vi "Control Experiment.vi"(8 "Error In":errorcluster, 9 "KH":T5={"KH #"=[0, 1, 2, 3, 4, 5, 6, 7, 8, 9, 10, 11, 12, 13, 14, 15], "KH Configuration"=[enum."SE+ (-gnd)", enum."SE+ (-gnd)", enum."Differential", enum."Differential", enum."SE+ (-gnd)", enum."Differential", enum."Differential", enum."SE+ (-gnd)", enum."Differential", enum."Differential", enum."SE+ (-gnd)", enum."SE+ (-gnd)", enum."Differential", enum."Ground", enum."Ground", enum."Ground"], "KH Gain"=[enum."1000x", enum."1000x", enum."1000x", enum."1000x", enum."1000x", enum."1000x", enum."1000x", enum."1000x", enum."1000x", enum."1000x", enum."1000x", enum."1000x", enum."1000x", enum."1000x", enum."1000x", enum."100x"], "KH Shunt Resistor"=[enum."Open", enum."Open", enum."Open", enum."5k Ohms", enum."Open", enum."Open", enum."5k Ohms", enum."Open", enum."Open", enum."5k Ohms", enum."Open", enum."Open", enum."50k Ohms", enum."Open", enum."Open", enum."Open"]}, 10 "Lockin":T7={"AI"=[1, 2, 3, 4, 5, 6, 7, 8, 9, 10, 11, 12, 13, 14, 15, 16], "Electrode"=["4", "5", "6", "7", "9", "11", "12", "13", "16", "17", "20", "21", "1", "", "", ""], "Label"=[12, 14, 15, 13, 10, 11, 9, 8, 4, 2, 1, 3, 6, 0, 0, 0], "Electrode Config"=[enum."Current", enum."Voltage (SE)", enum."Voltage (SE)", enum."Current", enum."Voltage (SE)", enum."Voltage (SE)", enum."Current", enum."Current", enum."Voltage (SE)", enum."Current", enum."Current", enum."Voltage (SE)", enum."Gate", enum."Voltage (SE)", enum."Voltage (SE)", enum."Voltage (SE)"]} {"Label" items=["", "I+", "I-", "V1+", "V1-", "dV1", "Vsg", "Vbg", "I2+", "I2-", "V2+", "V2-", "I3+", "I3-", "V3+", "V3-"]}) -> (0 "Error Out":errorcluster)   [LabVIEW 2019, in "Control Experiment.lvclass"]
doc: "Use this VI to help configure your experiment.\n1. Choose Pickering or Not Pickering\n2. Configure the Electrode control to show which electrode is connected to which lockin\n3. Choose a Label for each electrode to configure Krohn Hite amplifier automatically\n4. Easily set all Krohn Hite channels to be \"all ground\" or \"all differential\" mode\n5. Fill out information about you and your device in the lower left corner\n6. When you are finished, or when you want to update the amplifiers, click the \"CREATE OUTPUT\" button located in upper right. Clicking this button will set the amplifiers, Pickering switch (if you have one), and write information to a functional global variable that you can easily read from elsewhere in your program"
uses:
  Control Experiment.lvclass
  Typedefs/Instrument--enum.ctl
  <userlib>/LevyLab/Krohn Hite 7008/typedefs/Shunt-Enum.ctl
  Typedefs/KH Mode-enum.ctl
  <userlib>/LevyLab/Krohn Hite 7008/typedefs/Input Configuration-Enum.ctl
  <userlib>/LevyLab/Krohn Hite 7008/typedefs/Gain-Enum.ctl
  <userlib>/LevyLab/Krohn Hite 7008/typedefs/SetAll-Array.ctl
  <userlib>/LevyLab/Krohn Hite 7008/typedefs/SetAll-Cluster.ctl
  <userlib>/LevyLab/Krohn Hite 7008/typedefs/Channel-Enum.ctl
  <userlib>/LevyLab/Krohn Hite 7008/typedefs/Filter-Enum.ctl
  <userlib>/LevyLab/Krohn Hite 7008/typedefs/Coupling-Enum.ctl
  <userlib>/LevyLab/Instrument Framework/SMOs/Configuration/Configuration.lvclass
  Typedefs/UI Controls --cluster.ctl
  <userlib>/LevyLab/Instrument Framework/SMOs/Logger.PGSQL/Logger.PGSQL.lvclass
  C:/Program Files (x86)/National Instruments/LabVIEW 2019/vi.lib/JKI/JKI SMO/SMO/SMO.lvclass
  Control Experiment.lvclass/Control Experiment.ctl
  <userlib>/_MGI/File/MGI Create Directory Chain Behavior Enum.ctl
  Typedefs/Control Experiment JSON--cluster.ctl
  <userlib>/LevyLab/Krohn Hite 7008/Instrument.KH7008.lvclass/Instrument.KH7008.ctl
  23189d07-d529-447d-957d-13a42bf56e57.vi
  9a447b37-f4f5-4836-8e27-fdda23b4a061.vi
  <vilib>/JDP Science/JSONtext/Variant to JSON Text.vi
  <vilib>/regexp/Match Regular Expression.xnode
  <vilib>/JDP Science/JSONtext/LVClass Serializer/JSONtext LVClass Serializer.lvclass
  <userlib>/LevyLab/Krohn Hite 7008/Instrument.KH7008.lvclass
  <vilib>/JKI/JKI SMO/SMO/SMO.lvclass
  <userlib>/LevyLab/Lockin-Multichannel/Instrument.Lockin/Instrument.Lockin.lvclass
panel:
  out "KH Addresses":refnum<visa-resource-name>[](array[refnum])=["COM20", "COM14"] caption="KH Address[A,B,C,...]"
  in  "I'm Finished Taking Data!":bool
  out "Values have changed":bool=TRUE
  in  "Create Output":bool
  in  "OK":bool
  out "Control Experiment":refnum<class "Control Experiment.lvclass">
  in  "C.E.":refnum<class "Control Experiment.lvclass">
  in  "Tab Control":T1(tab)
  in  "Instrument Configuration":bool
  out "Instruments":string="    devices:\n    \n    1. 80x80um rectangle\n    2. hash: 200 horizontal and vertical lines 400nm apart\n    3. hash structures: 400, 200nm apart horizontal and vertical lines"
  in  "DC Coupled":bool=TRUE
  in  "Bandwidth Filter":bool=TRUE
  in  "AO Channels":u32=8
  in  "Gain":dbl[](array[numeric])=[1.0, 1.0, 1.0, 1.0, 1.0, 1.0, 1.0, 1.0, 1.0, 1.0, 1.0, 1.0, 1.0, 1.0, 1.0, 1.0]
  in  "AI Channels":u32=16
  in  "KH All Buttons":T8(radio)
  in  "Defualt Shunt Resistor":T4=enum."5k Ohms"
  in  "Description":string="    devices:\n    \n    1. 80x80um rectangle\n    2. hash: 200 horizontal and vertical lines 400nm apart\n    3. hash structures: 400, 200nm apart horizontal and vertical lines"
  in  "Sample (SAXXXX)":string="SA40178"
  in  "Device (YYYYMMDD)":string="20210125"
  in  "Instrument":T9=enum."MNK"
  in  "Username":string="Aditi"
  in  "non KH":T10 {"Labels 2" items=["", "I+", "I-", "V1+", "V1-", "dV1", "Vsg", "Vbg", "I2+", "I2-", "V2+", "V2-", "I3+", "I3-", "V3+", "V3-"]}
  in  "Ring":u16(ring)=2 items=["----Sweep Control----", "Sweep Control.vi", "Continuous B Sweep.vi", "----Transport----", "IV.vi", "IV_Sweep.vi", "Lockin_time.vi", "Lockin_Vsg.vi", "Lockin_sweep.vi", "Lockin_AIWFM_time.vi", "THz_TimeDelay.vi", "Sweep_AIWFM_time.vi"]
  in  "Open VI":bool
  in  "Open Lockin":bool
  in  "Default Path":path=path "C:/temp" caption="Default Path (Do not add your instrument name here)(Typ. G:\\My Drive\\ansom\\Data)"
  out "Comments":string="Device: \r  Device Name: SA40178.20210125\r  Computer: KHOLEK\r  User: Aditi\r  Instrument: MNK\r  Description: |\r        devices:\r        \r        1. 80x80um rectangle\r        2. hash: 200 horizontal and vertical lines 400nm apart\r        3. hash structures: 400, 200nm apart horizontal and vertical lines\r\rExperiment: \r  Time: 2021-02-22T11:02:02\r  Description: |\r\rSweep: \r- Loop1: [OFF, 0.000000]\r- Loop2: [OFF, 0.000000]\r- Loop3: [OFF, 0.000000]\r- Loop4: [OFF, 0.000000]\r\rWiring: \r- Electrode 4: Lockin 1, V2, KH1 Channel 1, SE+ (-gnd), 1000x, Open\r- Electrode 5: Lockin 2, V2, KH1 Channel 2, SE+ (-gnd), 1000x, Open\r- Electrode 6: Lockin 3, I2, KH1 Channel 3, Differential, 1000x, 5k Ohms\r- Electrode 7: Lockin 4, I2, KH1 Channel 4, Differential, 1000x, 5k Ohms\r- Electrode 9: Lockin 5, V2, KH1 Channel 5, SE+ (-gnd), 1000x, Open\r- Electrode 11: Lockin 6, I2, KH1 Channel 6, Differential, 1000x, 5k Ohms\r- Electrode 12: Lockin 7, I2, KH1 Channel 7, Differential, 1000x, 5k Ohms\r- Electrode 13: Lockin 8, V2, KH1 Channel 8, SE+ (-gnd), 1000x, Open\r- Electrode 16: Lockin 9, I-, KH2 Channel 1, Differential, 1000x, 5k Ohms\r- Electrode 17: Lockin 10, I+, KH2 Channel 2, Differential, 1000x, 5k Ohms\r- Electrode 20: Lockin 11, V1+, KH2 Channel 3, SE+ (-gnd), 1000x, Open\r- Electrode 21: Lockin 12, V1-, KH2 Channel 4, SE+ (-gnd), 1000x, Open\r- Electrode 1: Lockin 13, Vsg, KH2 Channel 5, Differential, 1000x, 50k Ohms\r\rLockin: \r  AO: \r  - AO 1: amp = 0.000 mV, DC = 0.000 mV, f = 1.00 Hz, phi = 0.00°, Triangle\r  - AO 2: amp = 0.000 mV, DC = 0.000 mV, f = 1.00 Hz, phi = 0.00°, Triangle\r  - AO 3: amp = 0.000 mV, DC = 0.000 mV, f = 1.00 Hz, phi = 0.00°, Triangle\r  - AO 4: amp = 0.000 mV, DC = 0.000 mV, f = 1.00 Hz, phi = 0.00°, Triangle\r  - AO 5: amp = 0.000 mV, DC = 0.000 mV, f = 1.00 Hz, phi = 0.00°, Triangle\r  - AO 6: amp = 10.000 mV, DC = 0.000 mV, f = 1.00 Hz, phi = 0.00°, Triangle\r  - AO 7: amp = 0.000 mV, DC = 0.000 mV, f = 1.00 Hz, phi = 0.00°, Triangle\r  - AO 8: amp = 0.000 mV, DC = 0.000 mV, f = 1.00 Hz, phi = 0.00°, Triangle\r  - AO 9: amp = 0.000 mV, DC = 0.000 mV, f = 1.00 Hz, phi = 0.00°, Triangle\r  - AO 10: amp = 10.000 mV, DC = 0.000 mV, f = 1.00 Hz, phi = 0.00°, Triangle\r  - AO 11: amp = 0.000 mV, DC = 0.000 mV, f = 1.00 Hz, phi = 0.00°, Triangle\r  - AO 12: amp = 0.000 mV, DC = 0.000 mV, f = 1.00 Hz, phi = 0.00°, Triangle\r  - AO 13: amp = 0.000 mV, DC = 0.000 mV, f = 1.00 Hz, phi = 0.00°, Sine\r  - AO 14: amp = 0.000 mV, DC = 0.000 mV, f = 1.00 Hz, phi = 0.00°, Sine\r  - AO 15: amp = 0.000 mV, DC = 0.000 mV, f = 1.00 Hz, phi = 0.00°, Sine\r  - AO 16: amp = 0.000 mV, DC = 0.000 mV, f = 1.00 Hz, phi = 0.00°, Sine\r  - AO 17: amp = 0.000 mV, DC = -0.000 mV, f = 1.00 Hz, phi = 0.00°, Sine\r  - AO 18: amp = 0.000 mV, DC = 0.000 mV, f = 1.00 Hz, phi = 0.00°, Sine\r  - AO 19: amp = 0.000 mV, DC = 0.000 mV, f = 1.00 Hz, phi = 0.00°, Sine\r  - AO 20: amp = 0.000 mV, DC = 0.000 mV, f = 1.00 Hz, phi = 0.00°, Sine\r  - AO 21: amp = 0.000 mV, DC = 0.000 mV, f = 1.00 Hz, phi = 0.00°, Sine\r  - AO 22: amp = 0.000 mV, DC = 0.000 mV, f = 1.00 Hz, phi = 0.00°, Sine\r  - AO 23: amp = 0.000 mV, DC = 0.000 mV, f = 1.00 Hz, phi = 0.00°, Sine\r  - AO 24: amp = 0.000 mV, DC = 0.000 mV, f = 1.00 Hz, phi = 0.00°, Sine\r  REF: \r  - Lockin 1: f = 1.00 Hz, phi = 0.00°, TC = 0.10 s, order = 2 \r  Sampling: \r  - Fs: 10000.000000\r  - N: 1000\r"
  out "Device Folder":path=path "D:/Data/MNK/SA40178.20210125" caption="(\\base path\\project\\device\\ )"
  out "JSON String":string="{\r\n    \"Device\":{\r\n        \"Device\":\"SA40178.20210125\",\r\n        \"User\":\"Aditi\",\r\n        \"Time\":\"2021-02-22T11:02:02\",\r\n        \"Computer Name\":\"KHOLEK\"\r\n    },\r\n    \"Wiring\":{\r\n        \"Lockin Ch\":[\r\n            1,\r\n            2,\r\n            3,\r\n            4,\r\n            5,\r\n            6,\r\n            7,\r\n            8,\r\n            9,\r\n            10,\r\n            11,\r\n            12,\r\n            13,\r\n            14,\r\n            15,\r\n            16\r\n        ],\r\n        \"KH Electrodes\":[\r\n            \"4\",\r\n            \"5\",\r\n            \"6\",\r\n            \"7\",\r\n            \"9\",\r\n            \"11\",\r\n            \"12\",\r\n            \"13\",\r\n            \"16\",\r\n            \"17\",\r\n            \"20\",\r\n            \"21\",\r\n            \"1\",\r\n            \"\",\r\n            \"\",\r\n            \"\"\r\n        ],\r\n        \"KH Labels\":[\r\n            \"V2\",\r\n            \"V2\",\r\n            \"I2\",\r\n            \"I2\",\r\n            \"V2\",\r\n            \"I2\",\r\n            \"I2\",\r\n            \"V2\",\r\n            \"I-\",\r\n            \"I+\",\r\n            \"V1+\",\r\n            \"V1-\",\r\n            \"Vsg\",\r\n            \"\",\r\n            \"\",\r\n            \"\"\r\n        ],\r\n        \"Other Electrodes\":[\r\n            \"4\",\r\n            \"5\",\r\n            \"6\",\r\n            \"7\",\r\n            \"9\",\r\n            \"11\",\r\n            \"12\",\r\n            \"13\",\r\n            \"16\",\r\n            \"17\",\r\n            \"20\",\r\n            \"21\",\r\n            \"1\",\r\n            \"\",\r\n            \"\",\r\n            \"\"\r\n        ],\r\n        \"Other Labels\":[\r\n            \"V2\",\r\n            \"V2\",\r\n            \"I2\",\r\n            \"I2\",\r\n            \"V2\",\r\n            \"I2\",\r\n            \"I2\",\r\n            \"V2\",\r\n            \"I-\",\r\n            \"I+\",\r\n            \"V1+\",\r\n            \"V1-\",\r\n            \"Vsg\",\r\n            \"\",\r\n            \"\",\r\n            \"\"\r\n        ]\r\n    }\r\n}"
  in  "Labels Strings":string[](array[string])=["", "I+", "I-", "V1+", "V1-", "dV1", "Vsg", "Vbg", "I2+", "I2-", "V2+", "V2-", "I3+", "I3-", "V3+", "V3-"]
  out "YAML example":string="description: This is a dummy dataset which mimics smFRET data.\n\nsetup:\n    ## Mandatory fields\n    num_pixels: 2                # using 2 detectors\n    num_spots: 1                 # a single confocal excitation\n    num_spectral_ch: 2           # donor and acceptor detection\n    num_polarization_ch: 1       # no polarization selection\n    num_split_ch: 1              # no beam splitter\n    modulated_excitation: False  # CW excitation, no modulation\n    lifetime: False              # no TCSPC in detection\n\n    ## Optional fields\n    excitation_wavelengths:      # List of excitation wavelenghts\n       - !!float 532e-9\n    excitation_cw:               # List of booleans, True if wavelength is CW\n       - True\n    detection_wavelengths:       # Nominal center wavelength for each for detection ch\n       - !!float 580e-9\n       - !!float 640e-9\n\nsample:\n  sample_name: describe the sample here\n  buffer_name: describe the buffer here\n  dye_names: 'Cy3B, ATTO647N'   # Comma separates names of fluorophores\n\nidentity:\n    author: Author Name\n    author_affiliation: Name of Research Institution\n\nprovenance:\n    filename: 'photon_data.hdf5'\n    software: Acquisition Software Name\n\nphoton_data:\n    timestamps_specs:\n        timestamps_unit: !!float 10e-9  # 10 ns\n    measurement_specs:\n        measurement_type: smFRET\n        detectors_specs:\n            spectral_ch1: [0]  # list of donor's detector IDs\n            spectral_ch2: [1]  # list of acceptor's detector IDs"
  in  "String":string
  # "SANDBOX:"
  # "Sample"
  # "Krohn Hite"
  # "Lockin"
  # "Lockin"
  # "Krohn Hite"
  # "Other"
  # "Device and Project Description"
  # "Instrument Configuration"
  # "Experiment VIs"
  # "Path Configuration"
  # "Use this VI to help configure your experiment.\n1. Configure the Electrode control to show which electrode is connected to which lockin\n2. Choose a Label for each electrode to configure Krohn Hite amplifier automatically\n3. Easily set all Krohn Hite channels to be \"all ground\" or \"all differential\" mode\n4. Fill out information about you and your device in the lower left corner\n5. When you are finished, or when you want to update the amplifiers, click the \"CREATE OUTPUT\" button located in upper right.\nClicking this button will set the amplifiers, Pickering switch (if you have one), and write information to a functional global variable that you can easily read from elsewhere in your program"
  # "If you want to have new labels for the \"Labels\" field you can type them here"
  # "The magic words are:\nI\nVsg\nVbg\ndV\nV"
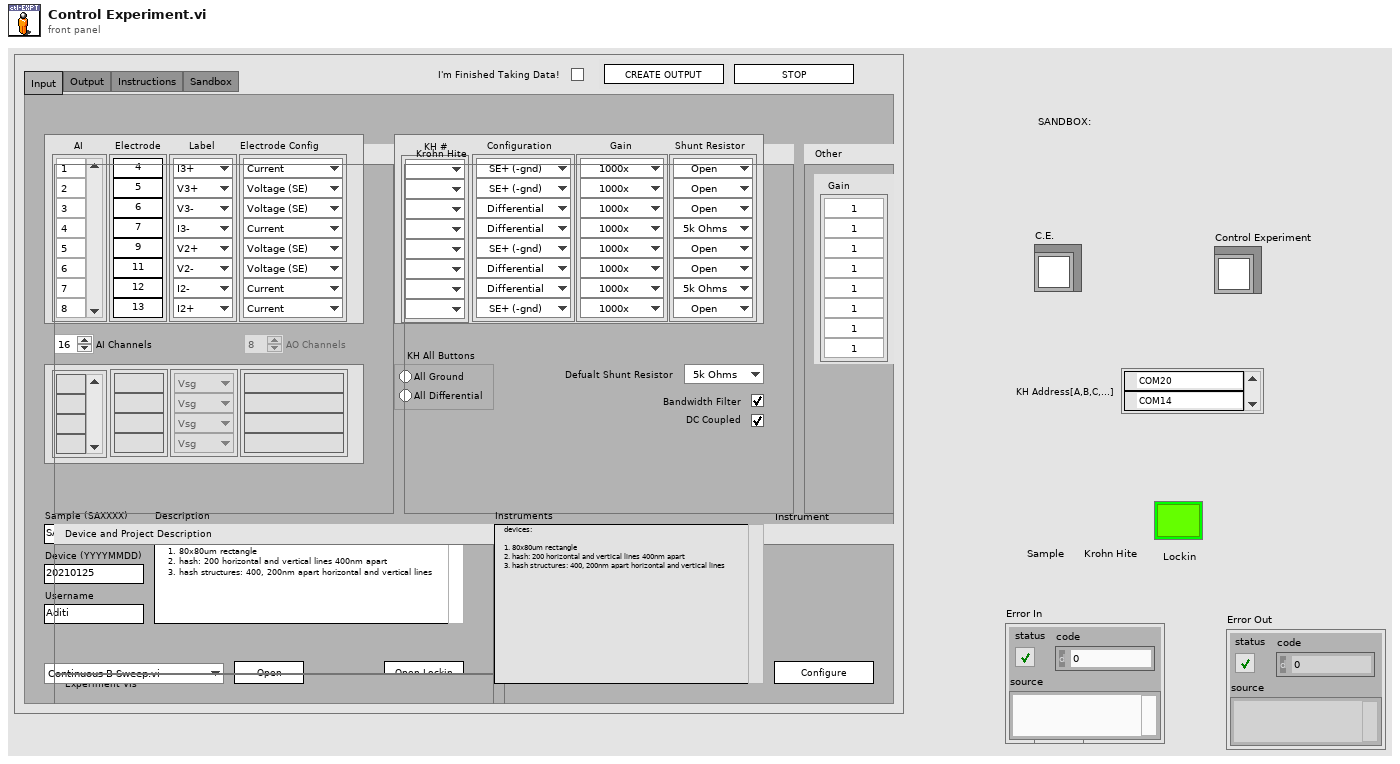
[diagram p1: front panel]
types:
  T1 = enum32{"Input", "Output", "Instructions", "Sandbox"}
  T2 = typedef "Instrument.KH7008.lvclass/Input Configuration-Enum.ctl" = enum16{"Ground", "SE+ (-gnd)", "SE- (+gnd)", "Differential"}
  T3 = typedef "Instrument.KH7008.lvclass/Gain-Enum.ctl" = enum16{"1x", "10x", "100x", "1000x"}
  T4 = typedef "Instrument.KH7008.lvclass/Shunt-Enum.ctl" = enum16{"Open", "50 Ohms", "500 Ohms", "5k Ohms", "50k Ohms", "10M Ohm"}
  T5 = cluster{"KH #":u16[], "KH Configuration":T2[], "KH Gain":T3[], "KH Shunt Resistor":T4[]}
  T6 = typedef "Control Experiment.lvclass/KH Mode-enum.ctl" = enum16{"Ground", "Current", "Voltage (SE)", "Voltage (Diff)", "Gate"}
  T7 = cluster{"AI":u32[], "Electrode":string[], "Label":u16[], "Electrode Config":T6[]}
  T8 = enum32{"No Selection", "All Ground", "All Differential"}
  T9 = typedef "Control Experiment.lvclass/Instrument--enum.ctl" = enum16{"----- AFM/EBL -----", "AGILENT", "CYPHER", "Gemini2", "JEOL", "MFP3D", "----- Cryostat -----", "CF900", "DR200", "MNK", "PPMS (simulated)", "PPMS 1", "PPMS 2", "PPMS 3", "----- Optics -----", "THz 1 (Element 2/Montana)", "THz 2 (Tsunami/Janis)"}
  T10 = cluster{"Scroll Bar":string[], "Electrodes 2":string[], "Labels 2":u16[], "unused":string[]}
  T11 = enum32{"invalid app kind", "Development System", "Run Time System", "Student Edition", "Embedded LabVIEW", "Evaluation", "Custom"}
  T12 = enum32{"Bad", "Idle", "Run top level", "Running"}
  T13 = enum32{"Invalid", "Standard", "Closed", "Hidden", "Minimized", "Maximized"}
  T14 = typedef "MGI Create Directory Chain Behavior Enum.ctl" = enum16{"Auto Detect", "Path Contains a File", "Path Does Not Contain a File"}
  T15 = typedef "Instrument.KH7008.lvclass/SetAll-Cluster.ctl" = cluster{"Channel":T16, "Gain":T3, "Bandwidth Filter":T17, "Shunt Resistor":T4, "Coupling":T18, "Input Config":T2}
  T16 = typedef "Instrument.KH7008.lvclass/Channel-Enum.ctl" = enum16{"Channel 1", "Channel 2", "Channel 3", "Channel 4", "Channel 5", "Channel 6", "Channel 7", "Channel 8"}
  T17 = typedef "Instrument.KH7008.lvclass/Filter-Enum.ctl" = enum16{"OFF", "ON"}
  T18 = typedef "Instrument.KH7008.lvclass/Coupling-Enum.ctl" = enum16{"AC", "DC"}
  T19 = typedef "Control Experiment.lvclass/Experiment Description--cluster.ctl" = cluster{"User":string, "Device":string, "Device Path":path, "Device Description":string, "Experiment Path":path, "Experiment Description":string, "Instrument":T9, "Instruments":cluster{"class path":path, "Address":string, "Type":T20}[], "Sweep":cluster{"key":string, "value":variant}[]}
  T20 = typedef "Control Experiment.lvclass/Instrument Types--combo.ctl" = string
  T21 = typedef "Control Experiment.lvclass/Wiring Description--cluster.ctl" = cluster{"Lockin Ch":i32[], "KH":cluster{"Electrodes":string[], "Labels":string[]}, "not KH":cluster{"Electrodes":string[], "Labels":string[]}}
  T22 = typedef "Instrument.KH7008.lvclass/SetAll-Array.ctl" = T15[]
  T23 = typedef "Control Experiment.lvclass/UI Controls --cluster.ctl" = cluster{"Sample":string, "Device":string, "Username":string, "Description":string, "Default Path":path, "AWS Path":path, "Instrument":T9, "Lockin?":bool, "Lockin Address":string, "Krohn Hite?":bool, "KH Addresses":refnum<visa-resource-name>[], "KH All Buttons":enum32{"No Selection", "All Ground", "All Differential"}, "Strain Cell?":bool, "Strain Cell Address":refnum<visa-resource-name>, "C Bridge?":bool, "Capacitance Bridge Address":refnum<visa-resource-name>, "Lockin":cluster{"AI":u32[], "Electrode":string[], "Label":u16[], "Electrode Config":T6[]}, "KH":cluster{"KH #":enum16{"A 1", "A 2", "A 3", "A 4", "A 5", "A 6", "A 7", "A 8", "B 1", "B 2", "B 3", "B 4", "B 5", "B 6", "B 7", "B 8", "none"}[], "KH Configuration":T2[], "KH Gain":T3[], "KH Shunt Resistor":T4[], "Filter":bool, "DC Coupled":bool}, "non KH":cluster{"Scroll Bar":string[], "Electrodes 2":string[], "Labels 2":u16[], "unused":string[]}}
  T24 = cluster{"Core":cluster{"Current VI Reference":refnum<vi>, "Close Panel on Exit?":bool}, "C.E.":refnum<class "Control Experiment.lvclass">, "Experiment":T19, "Wiring Configuration":T21, "Channel Settings":cluster{"Channel Setting":T22}[], "KH All Buttons":enum32{"No Selection", "All Ground", "All Differential"}, "Lockin":cluster{"AI":u32[], "Electrode":string[], "Label":u16[], "Electrode Config":T6[]}, "KH":cluster{"KH #":u16[], "KH Configuration":T2[], "KH Gain":T3[], "KH Shunt Resistor":T4[]}, "non KH":cluster{"Scroll Bar":string[], "Electrodes 2":string[], "Labels 2":u16[], "unused":string[]}, "UI":T23, "Logger":refnum<class "Logger.PGSQL.lvclass">, "Config":refnum<class "Configuration.lvclass">, "VI paths":path[], "top level?":bool}
  T25 = cluster{"Current VI Reference":refnum<vi>, "Close Panel on Exit?":bool}
  T26 = enum16{"A 1", "A 2", "A 3", "A 4", "A 5", "A 6", "A 7", "A 8", "B 1", "B 2", "B 3", "B 4", "B 5", "B 6", "B 7", "B 8", "none"}[]
  T27 = cluster{"class path":path, "Address":string, "Type":T20}[]
  T28 = typedef "Control Experiment.lvclass/Control Experiment JSON--cluster.ctl" = cluster{"Device":cluster{"Device":string, "User":string, "Time":string, "Computer Name":string}, "Wiring":cluster{"Lockin Ch":u32[], "KH Electrodes":string[], "KH Labels":string[], "Other Electrodes":string[], "Other Labels":string[]}}
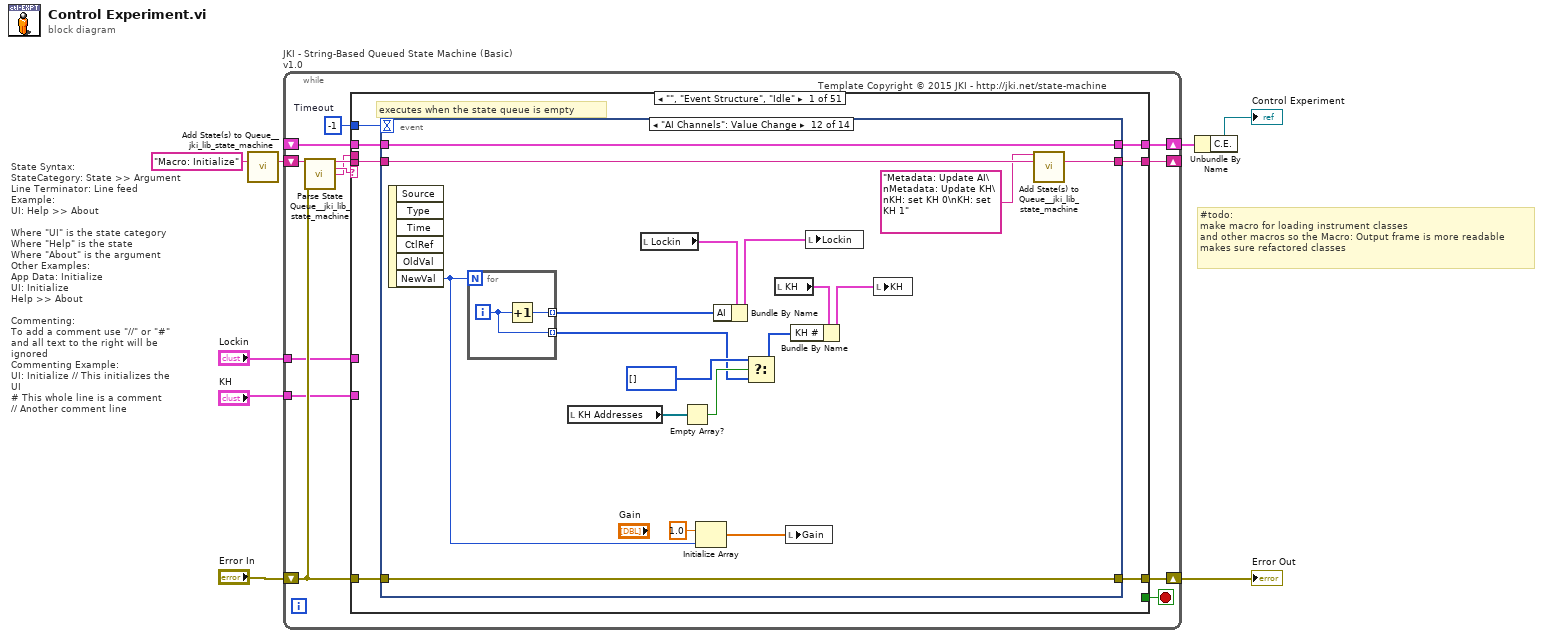
[diagram p0: block diagram]
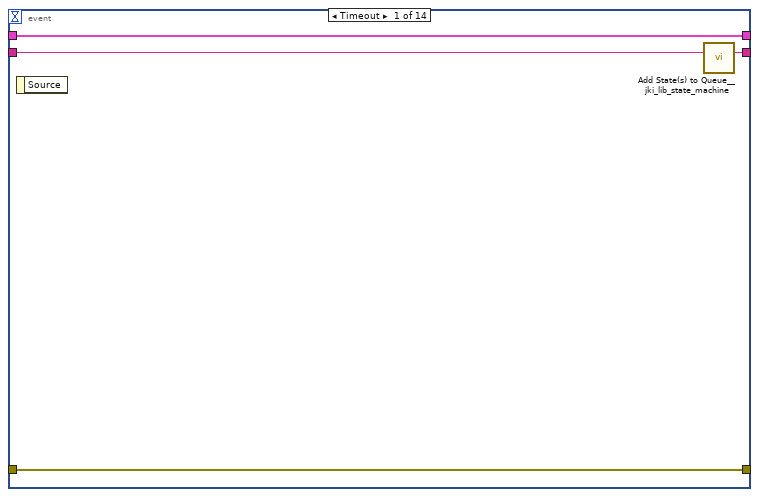
[diagram p2: hidden frame]
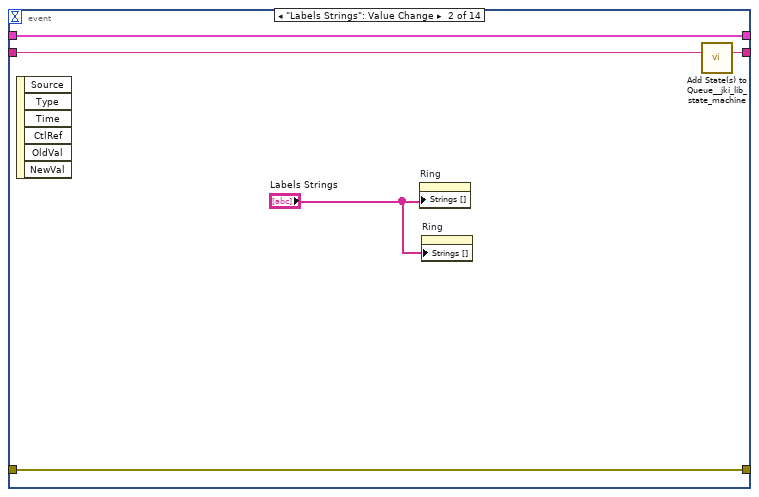
[diagram p3: hidden frame]
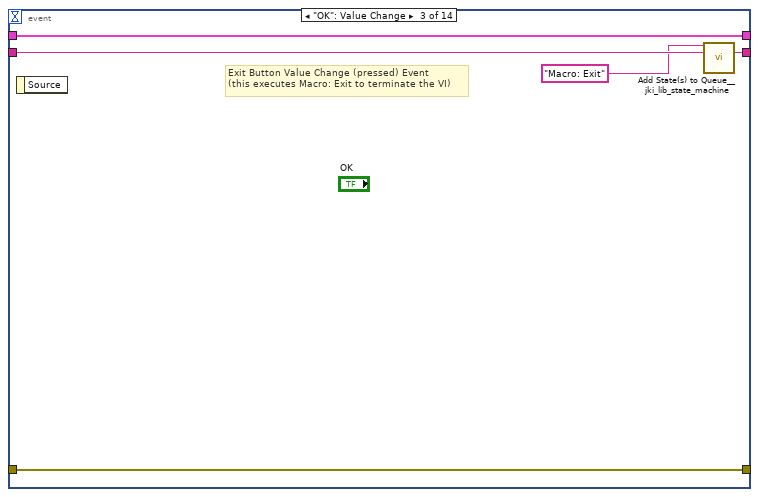
[diagram p4: hidden frame]
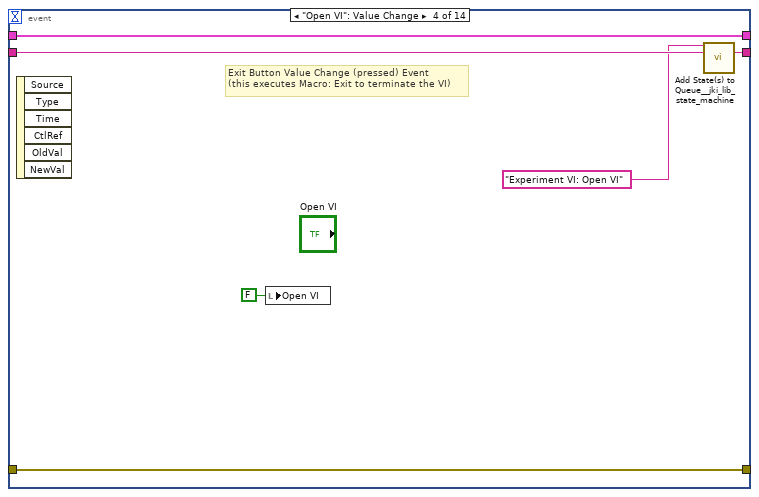
[diagram p5: hidden frame]
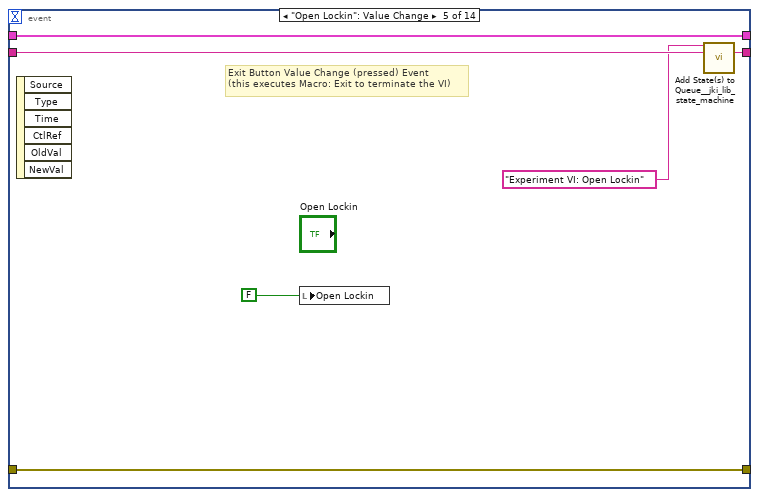
[diagram p6: hidden frame]
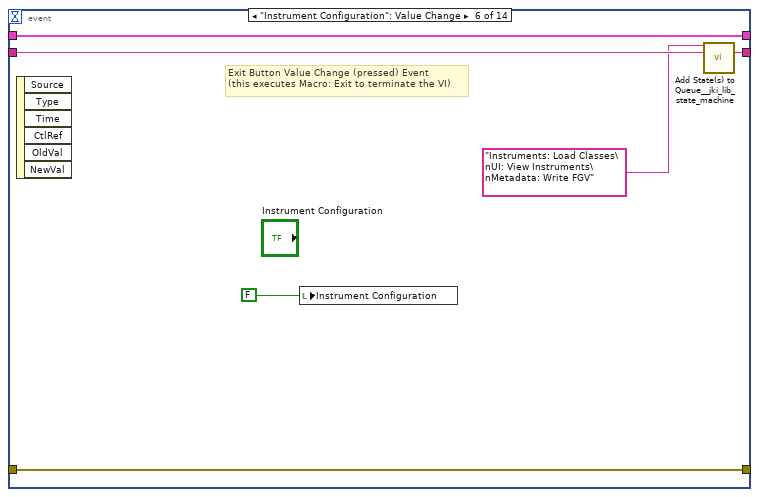
[diagram p7: hidden frame]
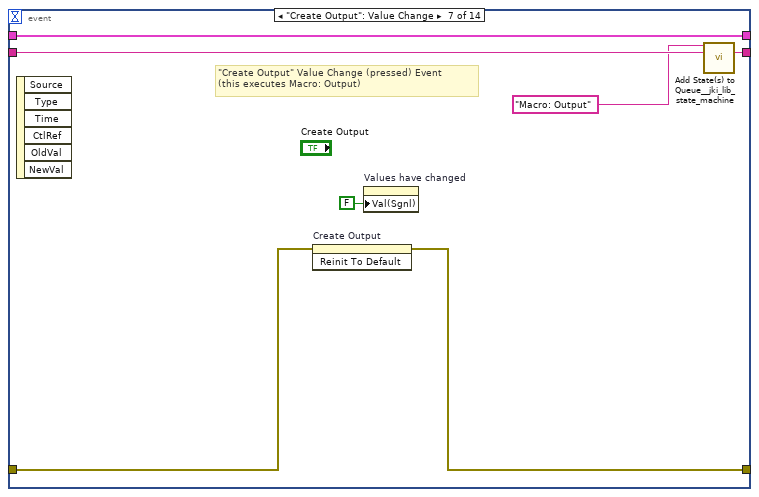
[diagram p8: hidden frame]
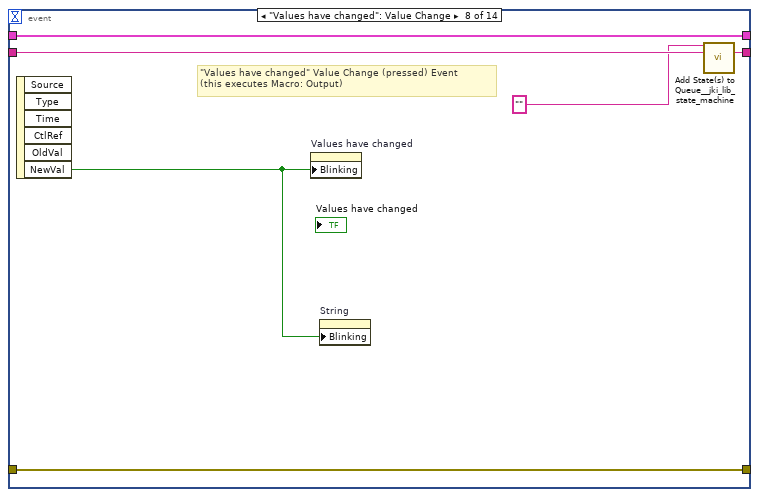
[diagram p9: hidden frame]
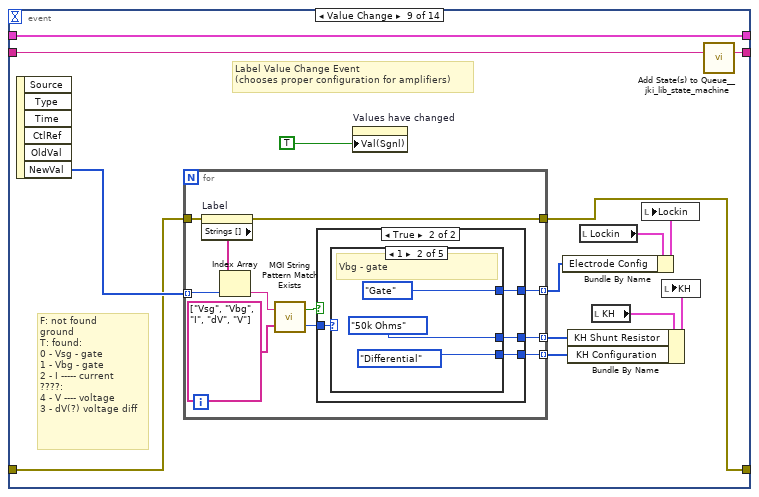
[diagram p10: hidden frame]
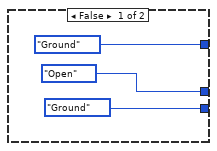
[diagram p11: hidden frame]
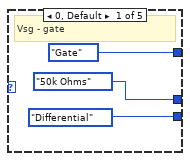
[diagram p12: hidden frame]
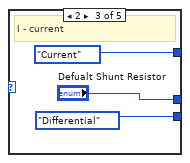
[diagram p13: hidden frame]
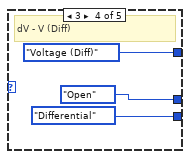
[diagram p14: hidden frame]
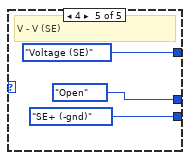
[diagram p15: hidden frame]
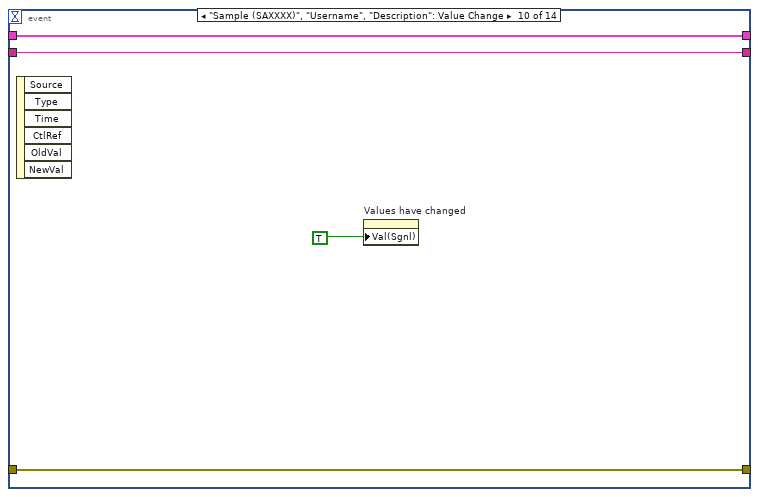
[diagram p16: hidden frame]
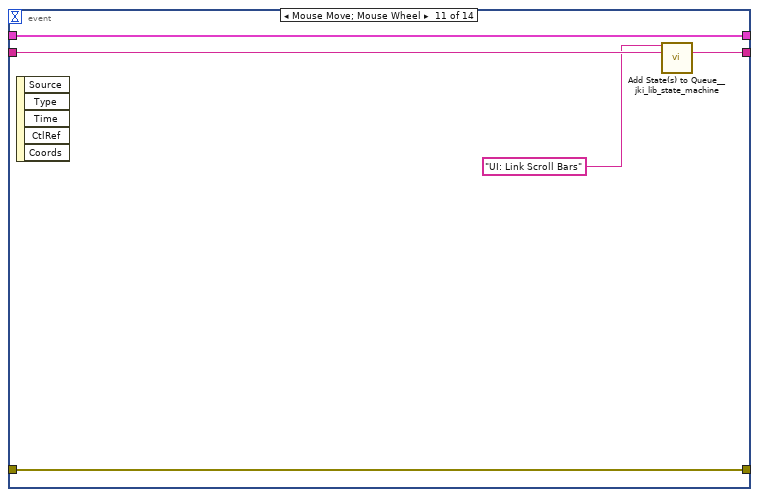
[diagram p17: hidden frame]
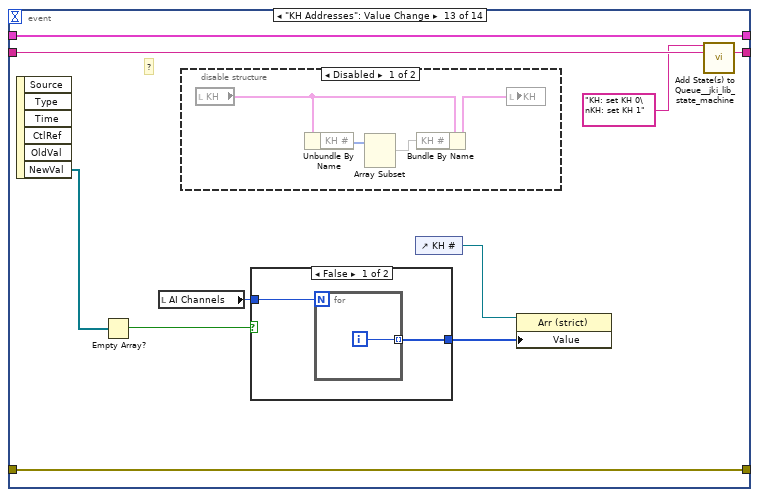
[diagram p18: hidden frame]
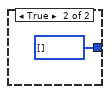
[diagram p20: hidden frame]
diagram:
  # "#todo:\nmake macro for loading instrument classes\nand other macros so the Macro: Output frame is more readable\nmakes sure refactored classes"
  # "State Syntax:\nStateCategory: State >> Argument\nLine Terminator: Line feed\nExample:\nUI: Help >> About\n\nWhere \"UI\" is the state category\nWhere \"Help\" is the state\nWhere \"About\" is the argument\nOther Examples:\nApp Data: Initialize\nUI: Initialize\nHelp >> About\n\nCommenting:\nTo add a comment use \"//\" or \"#\" and all text to the right will be ignored\nCommenting Example:\nUI: Initialize // This initializes the UI\n# This whole line is a comment\n// Another comment line"
  n1 = call <vilib>:"Add State(s) to Queue__jki_lib_state_machine.vi"("State(s) in (\"\")"="Macro: Initialize") -> ("States Out"=w8:string)  [unwired: 14 in]
  n2 = while "JKI - String-Based Queued State Machine (Basic) v1.0" {
    shift-right: [w14] -> w6
    shift-left: _ -> [w13]
    shift-right: [w17] -> w2
    shift-left: "Error In" -> [w11]
    shift-right: [w16] -> _
    shift-left: w8 -> [w18]
    tunnel: "Lockin" -> [w10]
    tunnel: "KH" -> [w9]
    stop <- w15 stop-if-true
    w12 = -1  # Timeout
    # "Template Copyright © 2015 JKI - http://jki.net/state-machine"
    n3 = call <vilib>:"Parse State Queue__jki_lib_state_machine.vi"("State Queue"=w18, "Error In (no error)"=w11) -> ("Remaining States"=w20:string, "Current State"=w21:string, "Arguments"=w19:string)  [unwired: 11 in]
    n4 = case shown="\"\", \"Event Structure\", \"Idle\"" w21 {
      selector: w21 -> [_ _ w178 _ _ _ _ _ _ _ _ _ _ _ _ _ _ _ _ _ _ _ _ _ _ _ _ _ _ _ _ _ _ _ _ _ _ _ _ _ _ _ _ _ _ _ _ _ _ _ _]
      tunnel: w20 -> [w28 w177 w182 w200 w206 w211 w215 w233 w244 w259 w285 w295 w299 w312 w337 w349 w362 w373 w399 w414 w427 w431 w436 w447 w454 w467 w472 w476 w488 w504 w528 w587 w646 w769 w782 w789 w797 w819 w823 w840 w879 w966 w981 w991 w1005 w1026 w1040 w1045 w1049 w1059 w1077]
      tunnel: w19 -> [_ _ _ _ _ _ _ _ _ _ _ _ _ _ _ _ w357 w367 _ _ _ _ _ _ _ _ _ _ _ _ _ _ _ _ _ _ _ _ _ _ _ _ _ _ _ _ _ _ _ _ _]
      tunnel: w13 -> [w26 w174 w180 w191 w203 w209 w212 _ w239 w255 w270 w290 w296 w302 w315 w346 w360 w369 w396 w411 w425 w428 w433 w444 w452 w464 w469 w473 w484 w500 w526 w585 w644 w765 w780 w787 w790 w813 w820 w838 w871 w959 w978 w989 w1002 w1013 w1038 w1043 w1046 w1051 w1075]
      tunnel: [w25 w175 w184 w197 errorcluster {"status"=FALSE, "code"=0, "source"=""} ("error out") w208 w213 w230 w242 w250 w271 w293 w297 w303 w335 w341 w358 w370 w397 w412 w415 w429 w434 w445 w450 w465 w470 w474 w486 w502 w519 w580 w637 w762 w770 w784 w794 w808 w821 w829 w870 w963 w979 w986 w1003 w1024 w1033 w1041 w1047 w1052 w1063] -> w17
      tunnel: w11 -> [w24 w175 w183 w197 w202 w208 w213 w230 w242 w256 w272 w291 w297 w310 w335 w341 w359 w371 w397 w412 w422 w429 w434 w445 w450 w465 w470 w474 w486 w502 w516 w577 w638 w762 w771 w783 w793 w798 w821 w824 w870 w955 w979 w985 w1003 w1024 w1034 w1042 w1047 w1053 w1065]
      tunnel: [w27 w176 w181 w199 w205 w210 w214 w232 w243 w258 w284 w294 w298 w311 w336 w348 w361 w372 w398 w413 w426 w430 w435 w446 w453 w466 w471 w475 w487 w503 w527 w586 w645 w768 w781 w788 w796 w818 w822 w839 w878 w965 w980 w990 w1004 w1025 w1039 w1044 w1048 w1058 w1076] -> w16
      tunnel: [_ _ _ _ _ TRUE _ _ _ _ _ _ _ _ _ _ _ _ _ _ _ _ _ _ _ _ _ _ _ _ _ _ _ _ _ _ _ _ _ _ _ _ _ _ _ _ _ _ _ _ _] -> w15
      tunnel: [w23 w174 w180 w198 w203 w209 w212 w231 w238 w254 w261 w290 w296 w302 w315 w346 w360 w369 w396 w411 w425 w428 w433 w444 w452 w464 w469 w473 w485 w501 w512 w571 w643 w764 w779 w787 w791 w813 w820 w837 w877 w964 w978 w988 w1002 w1012 w1038 w1043 w1046 w1050 w1075] -> w14
      tunnel: w12 -> [w22 _ _ _ _ _ _ _ _ _ _ _ _ _ _ _ _ _ _ _ _ _ _ _ _ _ _ _ _ _ _ _ _ _ _ _ _ _ _ _ _ _ _ _ _ _ _ _ _ _ _]
      tunnel: w10 -> [_ _ _ _ _ _ _ w217 _ _ _ _ _ _ _ _ _ _ _ _ _ _ _ _ _ _ _ _ _ _ _ _ _ _ _ _ _ _ _ _ _ _ _ _ _ _ _ _ _ _ _]
      tunnel: w9 -> [_ _ _ _ _ _ _ w216 _ _ _ _ _ _ _ _ _ _ _ _ _ _ _ _ _ _ _ _ _ _ _ _ _ _ _ _ _ _ _ _ _ _ _ _ _ _ _ _ _ _ _]
      frame "", "Event Structure", "Idle" {
        # "executes when the state queue is empty"
        n5 = event shown="[11] \"AI Channels\": Value Change" {
          selector: _ -> [_ _ _ _ _ _ _ _ _ _ _ _ _ _]
          dyn-events: _ -> [_ _ _ _ _ _ _ _ _ _ _ _ _ _]
          timeout: w22 -> [_ _ _ _ _ _ _ _ _ _ _ _ _ _]
          tunnel: w28 -> [w32 w35 w42 w48 w54 w60 w67 w73 w87 w122 w127 w146 w159 w173]
          tunnel: [w31 w37 w41 w47 w53 w59 w66 w72 w86 w122 w126 w145 w158 w172] -> w27
          tunnel: w26 -> [w29 w36 w39 w45 w51 w57 w65 w71 w85 w123 w128 w144 w156 w170]
          tunnel: [w30 w34 w40 w46 w52 w58 w62 w69 w74 w124 w129 w147 w157 w171] -> w25
          tunnel: w24 -> [w30 w34 w40 w46 w52 w58 w63 w69 w83 w124 w129 w147 w157 w171]
          tunnel: [w29 w36 w39 w45 w51 w57 w65 w71 w85 w123 w128 w144 w156 w170] -> w23
          event Timeout {
            n6 = event-data() -> ()  [unwired: 1 in, 1 out]
            n7 = call <vilib>:"Add State(s) to Queue__jki_lib_state_machine.vi"("State(s) in (\"\")"=w32) -> ("States Out"=w31:string)  [unwired: 14 in]
          }
          event "Labels Strings": Value Change {
            n8 = event-data() -> ()  [unwired: 1 in, 6 out]
            n9 = property on="Ring" class="Ring (strict)"("Strings []"="Labels Strings") -> ()  [unwired: 2 in, 2 out]
            n10 = property on="Ring" class="Ring (strict)"("Strings []"="Labels Strings") -> ()  [unwired: 2 in, 2 out]
            n11 = call <vilib>:"Add State(s) to Queue__jki_lib_state_machine.vi"("State(s) in (\"\")"=w35) -> ("States Out"=w37:string)  [unwired: 14 in]
          }
          event "OK": Value Change {
            # "Exit Button Value Change (pressed) Event\n(this executes Macro: Exit to terminate the VI)"
            n12 = event-data() -> ()  [unwired: 1 in, 1 out]
            n13 = call <vilib>:"Add State(s) to Queue__jki_lib_state_machine.vi"("State(s) in Front (\"\")"="Macro: Exit", "State(s) in (\"\")"=w42) -> ("States Out"=w41:string)  [unwired: 13 in]
          }
          event "Open VI": Value Change {
            # "Exit Button Value Change (pressed) Event\n(this executes Macro: Exit to terminate the VI)"
            n14 = event-data() -> ()  [unwired: 1 in, 6 out]
            n15 = local write "Open VI"(FALSE ("Open VI")) -> ()
            n16 = call <vilib>:"Add State(s) to Queue__jki_lib_state_machine.vi"("State(s) in Front (\"\")"="Experiment VI: Open VI", "State(s) in (\"\")"=w48) -> ("States Out"=w47:string)  [unwired: 13 in]
          }
          event "Open Lockin": Value Change {
            # "Exit Button Value Change (pressed) Event\n(this executes Macro: Exit to terminate the VI)"
            n17 = event-data() -> ()  [unwired: 1 in, 6 out]
            n18 = local write "Open Lockin"(FALSE ("Open VI")) -> ()
            n19 = call <vilib>:"Add State(s) to Queue__jki_lib_state_machine.vi"("State(s) in Front (\"\")"="Experiment VI: Open Lockin", "State(s) in (\"\")"=w54) -> ("States Out"=w53:string)  [unwired: 13 in]
          }
          event "Instrument Configuration": Value Change {
            # "Exit Button Value Change (pressed) Event\n(this executes Macro: Exit to terminate the VI)"
            n20 = event-data() -> ()  [unwired: 1 in, 6 out]
            n21 = local write "Instrument Configuration"(FALSE ("Open VI")) -> ()
            n22 = call <vilib>:"Add State(s) to Queue__jki_lib_state_machine.vi"("State(s) in Front (\"\")"="Instruments: Load Classes\nUI: View Instruments\nMetadata: Write FGV", "State(s) in (\"\")"=w60) -> ("States Out"=w59:string)  [unwired: 13 in]
          }
          event "Create Output": Value Change {
            # "\"Create Output\" Value Change (pressed) Event\n(this executes Macro: Output)"
            n23 = event-data() -> ()  [unwired: 1 in, 6 out]
            n24 = invoke on="Create Output" class="Bool" method="Reinit To Default"(error in=w63) -> (error out=w62:errorcluster)  [unwired: 2 in, 2 out]
            n25 = property on="Values have changed" class="Bool (strict)"("Val(Sgnl)"=FALSE ("Value (Signaling)")) -> ()  [unwired: 2 in, 2 out]
            n26 = call <vilib>:"Add State(s) to Queue__jki_lib_state_machine.vi"("State(s) in Front (\"\")"="Macro: Output", "State(s) in (\"\")"=w67) -> ("States Out"=w66:string)  [unwired: 13 in]
          }
          event "Values have changed": Value Change {
            # "\"Values have changed\" Value Change (pressed) Event\n(this executes Macro: Output)"
            n27 = event-data() -> ("NewVal"=w68:bool)  [unwired: 1 in, 5 out]
            n28 = property on="Values have changed" class="Bool (strict)"("Blinking"=w68) -> ()  [unwired: 2 in, 2 out]
            n29 = property on="String" class="Str"("Blinking"=w68) -> ()  [unwired: 2 in, 2 out]
            n30 = call <vilib>:"Add State(s) to Queue__jki_lib_state_machine.vi"("State(s) in Front (\"\")"="", "State(s) in (\"\")"=w73) -> ("States Out"=w72:string)  [unwired: 13 in]
          }
          event "Lockin.Label": Value Change {
            # "F: not found\nground\nT: found:\n0 - Vsg - gate\n1 - Vbg - gate\n2 - I ----- current\n????:\n4 - V ---- voltage\n3 - dV(?) voltage diff"
            # "Label Value Change Event\n(chooses proper configuration for amplifiers)"
            n31 = event-data() -> ("NewVal"=w84:u16[])  [unwired: 1 in, 5 out]
            n32 = for {
              tunnel: w84 -> [w95] mode=indexing
              tunnel: [w97] -> w79 mode=indexing
              tunnel: w83 -> [w94]
              tunnel: [w93] -> w74
              tunnel: [w92] -> w76 mode=indexing
              tunnel: [w88] -> w77 mode=indexing
              n33 = property on="Label" class="Ring (strict)"(error in=w94) -> (error out=w93:errorcluster, "Strings []"=w96:string[])  [unwired: 1 in, 1 out]
              n34 = Index Array(array=w96, index=w95) -> (element=w91:string)
              n35 = call <userlib>:"MGI String Pattern Match Exists.vi"("Patterns to Try"=string[] ["Vsg", "Vbg", "I", "dV", "V"], "String"=w91) -> ("Index of First Pattern Matched"=w98:i32, "Match Found"=w89:bool)
              n36 = case shown="True" w89 {
                tunnel: w98 -> [_ w105]
                tunnel: [KH_Mode-enum."Ground" ("Enum") w104] -> w97
                tunnel: [Shunt-Enum."Open" ("Shunt Resistor") w103] -> w92
                tunnel: [Input_Configuration-Enum."Ground" ("Input Configuation") w102] -> w88
                frame False {
                }
                frame True {
                  n37 = case shown="1" w105 {
                    tunnel: [KH_Mode-enum."Gate" ("Enum") KH_Mode-enum."Gate" ("Enum") KH_Mode-enum."Current" ("Enum") KH_Mode-enum."Voltage (Diff)" ("Enum") KH_Mode-enum."Voltage (SE)" ("Enum")] -> w104
                    tunnel: [Shunt-Enum."50k Ohms" ("Shunt Resistor") Shunt-Enum."50k Ohms" ("Shunt Resistor") "Defualt Shunt Resistor" Shunt-Enum."Open" ("Shunt Resistor") Shunt-Enum."Open" ("Shunt Resistor")] -> w103
                    tunnel: [Input_Configuration-Enum."Differential" ("Input Configuation") Input_Configuration-Enum."Differential" ("Input Configuation") Input_Configuration-Enum."Differential" ("Input Configuation") Input_Configuration-Enum."Differential" ("Input Configuation") Input_Configuration-Enum."SE+ (-gnd)" ("Input Configuation")] -> w102
                    frame 0, Default {
                      # "Vsg - gate"
                    }
                    frame 1 {
                      # "Vbg - gate"
                    }
                    frame 2 {
                      # "I - current"
                    }
                    frame 3 {
                      # "dV - V (Diff)"
                    }
                    frame 4 {
                      # "V - V (SE)"
                    }
                  }
                }
              }
            }
            n38 = property on="Values have changed" class="Bool (strict)"("Val(Sgnl)"=TRUE ("Values have changed")) -> ()  [unwired: 2 in, 2 out]
            n39 = local read "Lockin"() -> (w81:T7)
            n40 = Bundle By Name(cluster=w81, "Electrode Config"=w79) -> (w80:T7)
            n41 = local read "KH"() -> (w78:T5)
            n42 = Bundle By Name(cluster=w78, "KH Shunt Resistor"=w76, "KH Configuration"=w77) -> (w75:T5)
            n43 = local write "Lockin"(w80) -> ()
            n44 = local write "KH"(w75) -> ()
            n45 = call <vilib>:"Add State(s) to Queue__jki_lib_state_machine.vi"("State(s) in (\"\")"=w87) -> ("States Out"=w86:string)  [unwired: 14 in]
          }
          event "KH.KH Shunt Resistor", "KH.KH Gain", "non KH.Electrodes 2", "non KH.Labels 2", "Sample (SAXXXX)", "Username", "Description", "Lockin.Electrode": Value Change {
            n46 = event-data() -> ()  [unwired: 1 in, 6 out]
            n47 = property on="Values have changed" class="Bool (strict)"("Val(Sgnl)"=TRUE ("Values have changed")) -> ()  [unwired: 2 in, 2 out]
          }
          event "Lockin.AI", "non KH.Scroll Bar": Mouse Move; "Lockin.AI", "non KH.Scroll Bar": Mouse Wheel {
            n48 = event-data() -> ()  [unwired: 1 in, 5 out]
            n49 = call <vilib>:"Add State(s) to Queue__jki_lib_state_machine.vi"("State(s) in Front (\"\")"="UI: Link Scroll Bars" ("State(s) in Front (\"\")"), "State(s) in (\"\")"=w127) -> ("States Out"=w126:string)  [unwired: 13 in]
          }
          event "AI Channels": Value Change {
            n50 = event-data() -> ("NewVal"=w140:u32)  [unwired: 1 in, 5 out]
            n51 = for {
              N: w140 -> [_]
              tunnel: [w149] -> w135 mode=indexing
              tunnel: [w148] -> w131 mode=indexing
              i -> [w148]
              n52 = Increment(x=w148) -> (x+1=w149:i32)
            }
            n53 = local read "KH Addresses"() -> (w134:refnum<visa-resource-name>[])
            n54 = local read "Lockin"() -> (w143:T7)
            n55 = Empty Array?(array=w134) -> (empty?=w133:bool)
            n56 = Initialize Array(1.0 ("element"), w140) -> (w138:dbl[])
            n57 = Bundle By Name(cluster=w143, "AI"=w135) -> (w142:T7)
            n58 = Select(t=i32[] [], s=w133, f=w131) -> (s? t:f=w130:i32[])
            n59 = local read "KH"() -> (w137:T5)
            n60 = local write "Gain"(w138) -> ()
            n61 = Bundle By Name(cluster=w137, "KH #"=w130) -> (w141:T5)
            n62 = local write "Lockin"(w142) -> ()
            n63 = local write "KH"(w141) -> ()
            n64 = call <vilib>:"Add State(s) to Queue__jki_lib_state_machine.vi"("State(s) in Front (\"\")"="Metadata: Update AI\nMetadata: Update KH\nKH: set KH 0\nKH: set KH 1" ("State(s) in Front (\"\")"), "State(s) in (\"\")"=w146) -> ("States Out"=w145:string)  [unwired: 13 in]
          }
          event "KH Addresses": Value Change {
            # "?"
            n65 = event-data() -> ("NewVal"=w151:refnum<visa-resource-name>[])  [unwired: 1 in, 5 out]
            n66 = Empty Array?(array=w151) -> (empty?=w150:bool)
            n67 = local read "AI Channels"() -> (w152:u32)
            n68 = disable-structure shown="Disabled" {
              frame Disabled {
                n69 = local read "KH"() -> (w160:T5)
                n70 = Unbundle By Name(w160) -> ("KH #"=w162:u16[])
                n71 = Array Subset(array=w162) -> (w161:u16[])  [unwired: 2 in]
                n72 = Bundle By Name(cluster=w160, "KH #"=w161) -> (w163:T5)
                n73 = local write "KH"(w163) -> ()
              }
              frame Enabled {
              }
            }
            n74 = case shown="False" w150 {
              tunnel: [w164 i32[] []] -> w153
              tunnel: w152 -> [w165 _]
              frame False {
                n75 = for {
                  N: w165 -> [_]
                  tunnel: [w166] -> w164 mode=indexing
                  i -> [w166]
                }
              }
              frame True {
              }
            }
            n76 = control-ref of="KH #"() -> (w154:refnum<vi>)
            n77 = property class="Arr (strict)"(reference=w154, "Value"=w153) -> ()  [unwired: 1 in, 2 out]
            n78 = call <vilib>:"Add State(s) to Queue__jki_lib_state_machine.vi"("State(s) in Front (\"\")"="KH: set KH 0\nKH: set KH 1", "State(s) in (\"\")"=w159) -> ("States Out"=w158:string)  [unwired: 13 in]
          }
          event Panel Close? {
            # "Discard the event because we'll close the front panel ourselves in Macro: Exit"
            # "Close Panel button (pressed) Event\n(this executes Macro: Exit to terminate the VI)"
            n79 = event-data() -> ()  [unwired: 1 in, 1 out]
            n80 = event-data("Discard?"=TRUE) -> ()  [unwired: 1 in, 1 out]
            n81 = call <vilib>:"Add State(s) to Queue__jki_lib_state_machine.vi"("State(s) in Front (\"\")"="Macro: Exit", "State(s) in (\"\")"=w173) -> ("States Out"=w172:string)  [unwired: 13 in]
          }
        }
      }
      frame "---------- Core ----------" {
        # "Do not put any code in this frame.\n(it is a separator no-op)"
        n82 = call <vilib>:"Add State(s) to Queue__jki_lib_state_machine.vi"("State(s) in (\"\")"=w177) -> ("States Out"=w176:string)  [unwired: 14 in]
      }
      frame Default {
        w187 = 42 items=["No error", "Argument error", "Memory is full", "Out of zone", "End of file", "File already open", "Generic file I/O error", "File not found", "File permission error", "Disk is full", "Duplicate path", "Too many files open", "System feature not enabled", "Resource file not found", "Cannot add resource", "Resource not found", "Image not found", "Image memory error", "Pen does not exist", "Config type invalid", "Config token not found", "Config parse error", "Config memory error", "Bad external code format", "Bad external code offset", "External code not present", "Null window", "Destroy window error", "Null menu", "Print aborted", "Bad print record", "Print driver error", "Windows error during printing", "Memory error during printing", "Print dialog error", "Generic print error", "Invalid device refnum", "Device not found", "Device parameter error", "Device unit error", "Cannot open device", "Device call aborted", "Generic error", "Cancelled by user", "Object ID too low", "Object ID too high", "Object not in heap", "Unknown heap", "Unknown object (invalid DefProc)", "Unknown object (DefProc not in table)", "Message out of range", "Invalid (null) method", "Unknown message", "Manager call not supported", "Bad address", "Network operation in progress", "Network operation timed out", "Connection is busy", "Network attribute not supported", "Network error", "Address in use", "System out of memory", "Connection aborted", "Connection refused", "Not connected", "Already connected", "Connection closed", "Initialization error (interapplication manager)", "Bad occurrence", "Wait on unbound occurrence handler", "Occurrence queue overflow", "Datalog type conflict", "Unused", "Unrecognized type (interapplication manager)", "Memory corrupt", "Failed to make temporary DLL", "Old CIN version", "Drag socket not found", "Failed to load drop-object", "Failed to register OLE object", "Failed to release OLE object", "Format specifier type mismatch", "Unknown format specifier", "Too few format specifiers", "Too many format specifiers", "Scan failed", "Newer CIN version", "Error converting to variant", "Runtime menu error", "Password tampered", "Variant attribute not found", "Incompatible variant data type", "Event data is not available", "Event Store is not present", "Occurrence is not found", "Event Queue is not created", "Event info is not available", "Refnum passed is NULL", "Error retrieving Class GUID", "Error retrieving CoClass GUID", "Error retrieving TypeLib GUID.", "Bad built application magic bytes.", "Specific driver is different from the specific driver associated with the Logical Name.", "There is no session opened to the class driver.", "Max Error", "MAX - Error with config objects", "MAX - Error loading configuration", "MAX - Group not supported"]
        # "Current State"
        # "Do not delete, rename, or modify this frame.\n(this is used to capture unhandled states and typos)"
        # "Handle mistyped state name (developer tool)"
        n83 = Format Into String(format string="Software Exception: Unhandled State \"%s\"." ("message"), error in=w183, w178) -> (resulting string=w186:string, error out=w185:errorcluster)  [unwired: 1 in]
        n84 = call <vilib>:"Error Cluster From Error Code.vi"("show call chain? (False)"=TRUE, "error in (no error)"=w185, "error message (\"\")"=w186, "error code (0)"=w187) -> ("error out"=w184:errorcluster)  [unwired: 5 in]
        n85 = call <vilib>:"Add State(s) to Queue__jki_lib_state_machine.vi"("State(s) in (\"\")"=w182) -> ("States Out"=w181:string)  [unwired: 14 in]
      }
      frame "Initialize Core Data" {
        # "Do not delete, rename, or modify this frame.\n(this is used to determine panel behavior on exit)"
        # "originally closed?"
        # "exe?"
        # "If panel starts closed or is an EXE, then close it when we exit"
        n86 = property class="VI"() -> ("Front Panel.Open"=w196:bool)  [unwired: 2 in, 2 out]
        n87 = property class="App"() -> ("App.Kind"=w195:T11)  [unwired: 2 in, 2 out]
        n88 = control-ref of="Current VI Reference"() -> (w189:refnum<vi>)
        n89 = Not(x=w196) -> (.not. x?=w193:bool)
        n90 = Equal?(x=w195, y=T11."Run Time System" ("Application:Kind")) -> (x = y?=w192:bool)
        n91 = Or(x=w193, y=w192) -> (x .or. y?=w190:bool)
        n92 = Bundle By Name(cluster=w191, "Core.Current VI Reference"=w189, "Core.Close Panel on Exit?"=w190) -> (w198:T24)
        n93 = call <vilib>:"Add State(s) to Queue__jki_lib_state_machine.vi"("State(s) in (\"\")"=w200) -> ("States Out"=w199:string)  [unwired: 14 in]
      }
      frame "Error Handler" {
        # "Unhandled Error -- Display it"
        # "Handle any errors here.\nYou can also output any states to clean-up after errors occur"
        # "Clear error"
        n94 = call <vilib>:"General Error Handler.vi"("error in (no error)"=w202) -> ()  [unwired: 10 in, 5 out]
        n95 = call <vilib>:"Add State(s) to Queue__jki_lib_state_machine.vi"("State(s) in Front (\"\")"="/* Post Error States", "State(s) in (\"\")"=w206) -> ("States Out"=w205:string)  [unwired: 13 in]
      }
      frame "Exit" {
        # "Do not put any code in this frame.\n(No errors that occur here will be handled.)"
        n96 = call <vilib>:"Add State(s) to Queue__jki_lib_state_machine.vi"("State(s) in (\"\")"=w211) -> ("States Out"=w210:string)  [unwired: 14 in]
      }
      frame "---------- Data ----------" {
        # "Do not put any code in this frame.\n(It is a separator no-op. You can make a copy of this frame to create a new Data frame)"
        n97 = call <vilib>:"Add State(s) to Queue__jki_lib_state_machine.vi"("State(s) in (\"\")"=w215) -> ("States Out"=w214:string)  [unwired: 14 in]
      }
      frame "Data: Initialize" {
        w218 = FALSE  # top level?
        w219 = path[] []  # VI paths
        w220 = refnum<class "Logger.PGSQL.lvclass"> refnum  # Logger
        w221 = T23 {"Sample"="", "Device"="", "Username"="", "Description"="", "Default Path"=path "", "AWS Path"=path "", "Instrument"=enum."----- AFM/EBL -----", "Lockin?"=FALSE, "Lockin Address"="", "Krohn Hite?"=FALSE, "KH Addresses"=[], "KH All Buttons"=enum."No Selection", "Strain Cell?"=FALSE, "Strain Cell Address"="", "C Bridge?"=FALSE, "Capacitance Bridge Address"="", "Lockin"={"AI"=[], "Electrode"=[], "Label"=[], "Electrode Config"=[]}, "KH"={"KH #"=[], "KH Configuration"=[], "KH Gain"=[], "KH Shunt Resistor"=[], "Filter"=FALSE, "DC Coupled"=FALSE}, "non KH"={"Scroll Bar"=[], "Electrodes 2"=[], "Labels 2"=[], "unused"=[]}}  # UI
        w225 = refnum<class "Configuration.lvclass"> refnum  # Config
        w227 = cluster{"Channel Setting":T22}[] []  # Channel Settings
        w223 = T25 {"Current VI Reference"=refnum, "Close Panel on Exit?"=FALSE}  # Core
        # "Initialize the shift-register data, here.\n(data names are defined by what you wire into the bundle function)"
        n98 = Unbundle By Name("C.E.") -> ("Experiment"=w228:T19, "Wiring Configuration"=w229:T21)
        n99 = Bundle("Core"=w223, "C.E."="C.E.", "Experiment"=w228, "Wiring Configuration"=w229, "Channel Settings"=w227, "KH All Buttons"="KH All Buttons", "Lockin"=w217, "KH"=w216, "non KH"="non KH", "UI"=w221, "Logger"=w220, "Config"=w225, "VI paths"=w219, "top level?"=w218) -> (w231:T24)  [unwired: 1 in]
        n100 = call <vilib>:"Add State(s) to Queue__jki_lib_state_machine.vi"("State(s) in (\"\")"=w233) -> ("States Out"=w232:string)  [unwired: 14 in]
      }
      frame "Data: Initialize Top Level" {
        # "Do not put any code in this frame.\n(It is a separator no-op. You can make a copy of this frame to create a new Data frame)"
        n101 = property class="VI"() -> ("Exec.State"=w241:T12)  [unwired: 2 in, 2 out]
        n102 = Equal?(x=w241, y=T12."Run top level" ("Execution:State")) -> (x = y?=w237:bool)
        n103 = Select(t="", s=w237, f="Macro: Output\nMacro: Exit") -> (s? t:f=w236:string)
        n104 = Bundle By Name(cluster=w239, "top level?"=w237) -> (w238:T24)
        n105 = call <vilib>:"Add State(s) to Queue__jki_lib_state_machine.vi"("State(s) in (\"\")"=w244, "State(s) at Back (\"\")"=w236) -> ("States Out"=w243:string)  [unwired: 13 in]
      }
      frame "Data: Load Configuration" {
        n106 = Unbundle By Name(w255) -> ("Config"=w257:refnum<class "Configuration.lvclass">, "UI"=w249:T23)
        n107 = call <userlib>:"Default Path.vi"("error in (no error)"=w256, "Folder Name [Application Name]"="Control Experiment" ("name or relative path"), "Configuration in"=w257) -> ("error out"=w252:errorcluster, "Configuration out"=w253:refnum<class "Configuration.lvclass">)  [unwired: 7 in]
        n108 = call <userlib>:"Read Configuration.vi"("INI Fomatted Cluster Type"=w249, "error in (no error)"=w252, "Configuration in"=w253) -> ("error out"=w251:errorcluster, "Configuration"=w247:variant, "Configuration out"=w248:refnum<class "Configuration.lvclass">)  [unwired: 6 in]
        n109 = Variant To Data(error in=w251, type=w249, Variant=w247) -> (data=w245:T23, error out=w250:errorcluster)
        n110 = Bundle By Name(cluster=w255, "Config"=w248, "UI"=w245) -> (w254:T24)
        n111 = call <vilib>:"Add State(s) to Queue__jki_lib_state_machine.vi"("State(s) in (\"\")"=w259) -> ("States Out"=w258:string)  [unwired: 14 in]
      }
      frame "Data: Save Controls" {
        n112 = local read "Sample (SAXXXX)"() -> (w283:string)
        n113 = local read "Lockin"() -> (w275:T7)
        n114 = local read "Username"() -> (w281:string)
        n115 = local read "Default Path"() -> (w279:path)
        n116 = local read "KH Addresses"() -> (w277:refnum<visa-resource-name>[])
        n117 = local read "KH"() -> (w268:T5)
        n118 = local read "Description"() -> (w280:string)
        n119 = Unbundle By Name(w268) -> ("KH #"=w267:u16[], "KH Configuration"=w264:T2[], "KH Gain"=w265:T3[], "KH Shunt Resistor"=w266:T4[])
        n120 = local read "Instrument"() -> (w278:T9)
        n121 = local read "Device (YYYYMMDD)"() -> (w282:string)
        n122 = local read "KH All Buttons"() -> (w276:T8)
        n123 = local read "non KH"() -> (w269:T10)
        n124 = Bundle By Name(cluster=w270, "UI.Sample"=w283, "UI.Device"=w282, "UI.Username"=w281, "UI.Description"=w280, "UI.Default Path"=w279, "UI.AWS Path"=path "", "UI.Instrument"=w278, "UI.KH Addresses"=w277, "UI.KH All Buttons"=w276, "UI.Lockin"=w275, "UI.non KH"=w269, "UI.KH.KH #"=w267, "UI.KH.KH Configuration"=w264, "UI.KH.KH Gain"=w265, "UI.KH.KH Shunt Resistor"=w266, "UI.KH.Filter"="Bandwidth Filter", "UI.KH.DC Coupled"="DC Coupled") -> (w261:T24)
        n125 = Unbundle By Name(w261) -> ("Config"=w274:refnum<class "Configuration.lvclass">, "UI"=w273:T23)
        n126 = call <userlib>:"Write Configuration.vi"("error in (no error)"=w272, "Variant"=w273, "Configuration in"=w274) -> ("error out"=w271:errorcluster)  [unwired: 7 in, 1 out]
        n127 = call <vilib>:"Add State(s) to Queue__jki_lib_state_machine.vi"("State(s) in (\"\")"=w285) -> ("States Out"=w284:string)  [unwired: 14 in]
      }
      frame "Data: Cleanup" {
        # "Cleanup any data and references, here.\n(this is called automatically, by the Macro: Exit)"
        n128 = Unbundle By Name(w290) -> ("Core.Current VI Reference"=w289:refnum<vi>, "Logger"=w292:refnum<class "Logger.PGSQL.lvclass">)
        n129 = call <vilib>:"Stop.vi"("error in (no error)"=w291, "SMO"=w292) -> ("error out"=w287:errorcluster, "SMO out"=w288:refnum<class "Logger.PGSQL.lvclass">)  [unwired: 8 in]
        n130 = call <vilib>:"Destroy.vi"("error in (no error)"=w287, "SMO"=w288) -> ("error out"=w286:errorcluster)  [unwired: 9 in]
        n131 = Close Reference(reference=w289, error in (no error)=w286) -> (error out=w293:errorcluster)
        n132 = call <vilib>:"Add State(s) to Queue__jki_lib_state_machine.vi"("State(s) in (\"\")"=w295) -> ("States Out"=w294:string)  [unwired: 14 in]
      }
      frame "---------- UI ----------" {
        # "Do not put any code in this frame.\n(It is a separator no-op. You can make a copy of this frame to create a new UI frame)"
        n133 = call <vilib>:"Add State(s) to Queue__jki_lib_state_machine.vi"("State(s) in (\"\")"=w299) -> ("States Out"=w298:string)  [unwired: 14 in]
      }
      frame "UI: Initialize" {
        (unwired) string[] ["", "I+", "I-", "V1+", "V1-", "V2+", "V2-", "V3+", "V3-", "V4+", "V4-", "dV1", "dV2", "dV3", "Vsg", "Vbg"] ("Strings [] 2")
        # "Initialize the User Interface, here.\n(this is called automatically, by the Macro: Init)"
        n134 = local read "Labels Strings"() -> (w306:string[])
        n135 = call <userlib>:"Fit VI window to Largest Dec__ogtk.vi"("error in (no error)"=w310) -> ("error out"=w308:errorcluster)  [unwired: 5 in, 1 out]
        n136 = Unbundle By Name(w302) -> ("top level?"=w300:bool)
        n137 = property on="OK" class="Bool (strict)"("Value"=FALSE ("Blinking")) -> ()  [unwired: 2 in, 2 out]
        n138 = property on="Tab Control" class="TabCtl (strict)"("Value"=T1."Input" ("Tab Control")) -> ()  [unwired: 2 in, 2 out]
        n139 = property on="Ring" class="Ring (strict)"(error in=w308, "Strings []"=w306) -> (error out=w307:errorcluster)  [unwired: 1 in, 1 out]
        n140 = local write "KH All Buttons"(T8."No Selection" ("KH All Buttons")) -> ()
        n141 = property on="Values have changed" class="Bool (strict)"("Val(Sgnl)"=TRUE ("Blinking")) -> ()  [unwired: 2 in, 2 out]
        n142 = property on="Ring" class="Ring (strict)"(error in=w307, "Strings []"=w306) -> (error out=w303:errorcluster)  [unwired: 1 in, 1 out]
        n143 = case shown="True" w300 {
          frame False {
          }
          frame True {
            # "unused"
            n144 = local read "KH Addresses"() -> (w313:refnum<visa-resource-name>[])
            n145 = property on="AI Channels" class="DigNum (strict)"("Val(Sgnl)"="AI Channels") -> ()  [unwired: 2 in, 2 out]
            n146 = property on="KH Addresses" class="Arr (strict)"("Val(Sgnl)"=w313) -> ()  [unwired: 2 in, 2 out]
          }
        }
        n147 = call <vilib>:"Add State(s) to Queue__jki_lib_state_machine.vi"("State(s) in (\"\")"=w312) -> ("States Out"=w311:string)  [unwired: 14 in]
      }
      frame "UI: Update Controls" {
        # "Do not put any code in this frame.\n(It is a separator no-op. You can make a copy of this frame to create a new Data frame)"
        n148 = Unbundle By Name(w315) -> ("top level?"=w316:bool, "UI.Sample"=w329:string, "UI.Device"=w330:string, "UI.Username"=w331:string, "UI.Description"=w332:string, "UI.Default Path"=w334:path, "UI.Instrument"=w333:T9, "UI.KH Addresses"=w328:refnum<visa-resource-name>[], "UI.KH All Buttons"=w327:T8, "UI.Lockin"=w318:T7, "UI.non KH"=w317:T10, "UI.KH.Filter"=w325:bool, "UI.KH.DC Coupled"=w326:bool, "UI.KH.KH #"=w322:T26, "UI.KH.KH Configuration"=w321:T2[], "UI.KH.KH Gain"=w320:T3[], "UI.KH.KH Shunt Resistor"=w319:T4[])  [unwired: 2 out]
        n149 = local write "Sample (SAXXXX)"(w329) -> ()
        n150 = local write "Username"(w331) -> ()
        n151 = local write "Instrument"(w333) -> ()
        n152 = local write "Default Path"(w334) -> ()
        n153 = local write "KH Addresses"(w328) -> ()
        n154 = local write "Bandwidth Filter"(w325) -> ()
        n155 = local write "DC Coupled"(w326) -> ()
        n156 = local write "Device (YYYYMMDD)"(w330) -> ()
        n157 = local write "Description"(w332) -> ()
        n158 = local write "KH All Buttons"(w327) -> ()
        n159 = local read "KH"() -> (w324:T5)
        n160 = Bundle By Name(cluster=w324, "KH #"=w322, "KH Configuration"=w321, "KH Gain"=w320, "KH Shunt Resistor"=w319) -> (w323:T5)
        n161 = case shown="True" w316 {
          tunnel: w323 -> [_ w340]
          tunnel: w318 -> [_ w339]
          tunnel: w317 -> [_ w338]
          frame False {
          }
          frame True {
            n162 = local write "non KH"(w338) -> ()
            n163 = local write "Lockin"(w339) -> ()
            n164 = local write "KH"(w340) -> ()
          }
        }
        n165 = call <vilib>:"Add State(s) to Queue__jki_lib_state_machine.vi"("State(s) in (\"\")"=w337) -> ("States Out"=w336:string)  [unwired: 14 in]
      }
      frame "UI: View Instruments" {
        n166 = Unbundle By Name(w346) -> ("C.E."=w347:refnum<class "Control Experiment.lvclass">)
        n167 = Unbundle By Name(w347) -> ("Instruments"=w345:T27)
        n168 = for {
          tunnel: w345 -> [w356] mode=indexing
          tunnel: [w350] -> w344 mode=indexing
          n169 = Unbundle By Name(w356) -> ("Type"=w353:T20, "class path"=w355:path, "Address"=w351:string)
          n170 = Strip Path(path=w355) -> (name=w352:string)  [unwired: 1 out]
          n171 = Format Into String(format string="%s:\n- %s\n- %s", w353, w352, w351) -> (resulting string=w350:string)  [unwired: 2 in, 1 out]
        }
        n172 = call <vilib>:"1D String Array to Delimited String.vi"("delimiter"="\n", "string array"=w344) -> ("delimited string"=→"Instruments":string)  [unwired: 9 in]
        n173 = call <vilib>:"Add State(s) to Queue__jki_lib_state_machine.vi"("State(s) in (\"\")"=w349) -> ("States Out"=w348:string)  [unwired: 14 in]
      }
      frame "UI: Cursor Set" {
        # "Argument"
        # "Set and Unset Cursor Busy.\n(Usage: \"UI: Cursor Set >> Busy|Idle\")"
        n174 = case shown="\"Busy\"" w357 {
          tunnel: w359 -> [w364 w366]
          tunnel: [w363 w365] -> w358
          frame "Idle", Default {
            n175 = call <vilib>:"Unset Busy.vi"("error in (no error)"=w364) -> ("error out"=w363:errorcluster)  [unwired: 10 in]
          }
          frame "Busy" {
            n176 = call <vilib>:"Set Busy.vi"("error in (no error)"=w366) -> ("error out"=w365:errorcluster)  [unwired: 9 in, 1 out]
          }
        }
        n177 = call <vilib>:"Add State(s) to Queue__jki_lib_state_machine.vi"("State(s) in (\"\")"=w362) -> ("States Out"=w361:string)  [unwired: 14 in]
      }
      frame "UI: Front Panel State" {
        # "Argument"
        # "Set Front Panel Open or Closed\n(Usage: \"UI: Front Panel State >> Open|Close\")"
        n178 = Unbundle By Name(w369) -> ("Core.Current VI Reference"=w368:refnum<vi>)
        n179 = case shown="\"Open\", Default" w367 {
          tunnel: w371 -> [w377 w390]
          tunnel: [w379 w391] -> w370
          tunnel: w368 -> [w378 w388]
          frame "Open", Default {
            n180 = property class="VI"(reference=w378, error in=w377) -> (reference out=w375:refnum<vi>, error out=w376:errorcluster, "Front Panel.Open"=w374:bool)
            n181 = case shown="True" w374 {
              tunnel: [w382 w385] -> w379
              tunnel: w376 -> [w381 w385]
              tunnel: w375 -> [w380 _]
              frame False {
                n182 = invoke class="VI" method="FP.Open"(reference=w380, error in=w381, "Activate"=TRUE, "State"=T13."Standard") -> (error out=w382:errorcluster)  [unwired: 1 in, 4 out]
              }
              frame True {
              }
            }
          }
          frame "Close" {
            n183 = property class="VI"(reference=w388, error in=w390) -> (reference out=w387:refnum<vi>, error out=w389:errorcluster, "Front Panel.Open"=w386:bool)
            n184 = case shown="True" w386 {
              tunnel: [w392 w395] -> w391
              tunnel: w389 -> [w392 w394]
              tunnel: w387 -> [_ w393]
              frame False {
              }
              frame True {
                n185 = invoke class="VI" method="FP.Close"(reference=w393, error in=w394) -> (error out=w395:errorcluster)  [unwired: 1 in, 2 out]
              }
            }
          }
        }
        n186 = call <vilib>:"Add State(s) to Queue__jki_lib_state_machine.vi"("State(s) in (\"\")"=w373) -> ("States Out"=w372:string)  [unwired: 14 in]
      }
      frame "UI: Buttons" {
        # "Do not put any code in this frame.\n(It is a separator no-op. You can make a copy of this frame to create a new UI frame)"
        n187 = call <vilib>:"Add State(s) to Queue__jki_lib_state_machine.vi"("State(s) in (\"\")"=w399) -> ("States Out"=w398:string)  [unwired: 14 in]
      }
      frame "UI: Link Scroll Bars" {
        # "Do not put any code in this frame.\n(It is a separator no-op. You can make a copy of this frame to create a new UI frame)"
        n188 = control-ref of="AI"() -> (w410:refnum<vi>)
        n189 = control-ref of="Electrode"() -> (w409:refnum<vi>)
        n190 = control-ref of="Label"() -> (w408:refnum<vi>)
        n191 = control-ref of="Electrode Config"() -> (w407:refnum<vi>)
        n192 = control-ref of="KH #"() -> (w406:refnum<vi>)
        n193 = control-ref of="KH Configuration"() -> (w405:refnum<vi>)
        n194 = control-ref of="KH Gain"() -> (w404:refnum<vi>)
        n195 = control-ref of="KH Shunt Resistor"() -> (w403:refnum<vi>)
        n196 = control-ref of="Gain"() -> (w401:refnum<vi>)
        n197 = property class="Arr (strict)"(reference=w410) -> ("Index Values"=w400:u32[])  [unwired: 1 in, 2 out]
        n198 = property class="Arr (strict)"(reference=w409, "Index Values"=w400) -> ()  [unwired: 1 in, 2 out]
        n199 = property class="Arr (strict)"(reference=w408, "Index Values"=w400) -> ()  [unwired: 1 in, 2 out]
        n200 = property class="Arr (strict)"(reference=w407, "Index Values"=w400) -> ()  [unwired: 1 in, 2 out]
        n201 = property class="Arr (strict)"(reference=w406, "Index Values"=w400) -> ()  [unwired: 1 in, 2 out]
        n202 = property class="Arr (strict)"(reference=w405, "Index Values"=w400) -> ()  [unwired: 1 in, 2 out]
        n203 = property class="Arr (strict)"(reference=w404, "Index Values"=w400) -> ()  [unwired: 1 in, 2 out]
        n204 = property class="Arr (strict)"(reference=w403, "Index Values"=w400) -> ()  [unwired: 1 in, 2 out]
        n205 = property class="Arr (strict)"(reference=w401, "Index Values"=w400) -> ()  [unwired: 1 in, 2 out]
        n206 = property on="Scroll Bar" class="Arr (strict)"() -> ("Index Values"=w402:u32[])  [unwired: 2 in, 2 out]
        n207 = property on="Labels 2" class="Arr (strict)"("Index Values"=w402) -> ()  [unwired: 2 in, 2 out]
        n208 = property on="unused" class="Arr (strict)"("Index Values"=w402) -> ()  [unwired: 2 in, 2 out]
        n209 = property on="Electrodes 2" class="Arr (strict)"("Index Values"=w402) -> ()  [unwired: 2 in, 2 out]
        n210 = call <vilib>:"Add State(s) to Queue__jki_lib_state_machine.vi"("State(s) in (\"\")"=w414) -> ("States Out"=w413:string)  [unwired: 14 in]
      }
      frame "UI: SR Disable" {
        # "Do not put any code in this frame.\n(It is a separator no-op. You can make a copy of this frame to create a new UI frame)"
        n211 = local read "KH Addresses"() -> (w424:refnum<visa-resource-name>[])
        n212 = control-ref of="Shunt Resistor"() -> (w420:refnum<vi>)
        n213 = Index Array(array=w424) -> (element=w423:refnum<visa-resource-name>)  [unwired: 1 in]
        n214 = call <userlib>:"Shunt - Check 500 or 10M.vi"("error in (no error)"=w422, "VISA Refnum in"=w423) -> ("error out"=w421:errorcluster, "SR"=w417:enum16{"500", "10M"})  [unwired: 7 in, 1 out]
        n215 = call <vilib>:"Clear Errors.vi"("error in (no error)"=w421) -> ("error out"=w419:errorcluster)  [unwired: 5 in, 1 out]
        n216 = call <userlib>:"Shunt - 500 or 10M Control Disable.vi"("error in"=w419, "SR"=w417, "reference"=w420) -> ("error out"=w416:errorcluster)  [unwired: 8 in]
        n217 = control-ref of="Defualt Shunt Resistor"() -> (w418:refnum<vi>)
        n218 = call <userlib>:"Shunt - 500 or 10M Control Disable.vi"("error in"=w416, "SR"=w417, "reference"=w418) -> ("error out"=w415:errorcluster)  [unwired: 8 in]
        n219 = call <vilib>:"Add State(s) to Queue__jki_lib_state_machine.vi"("State(s) in (\"\")"=w427) -> ("States Out"=w426:string)  [unwired: 14 in]
      }
      frame "---------- Macro ----------" {
        # "Do not put any code in this frame.\n(It is a separator no-op. You can make a copy of this frame to create a new Macro frame)"
        n220 = call <vilib>:"Add State(s) to Queue__jki_lib_state_machine.vi"("State(s) in (\"\")"=w431) -> ("States Out"=w430:string)  [unwired: 14 in]
      }
      frame "Macro: Initialize" {
        # "Initialization Macro\n(This is called once, when the VI starts)"
        n221 = call <vilib>:"Add State(s) to Queue__jki_lib_state_machine.vi"("State(s) in Front (\"\")"="Data: Initialize\nInitialize Core Data\nData: Initialize Top Level\nData: Load Configuration\nMetadata: Read FGV\nUI: View Instruments\nUI: Update Controls\nUI: Initialize\nUI: Front Panel State >> Open\nUI: SR Disable\nExperiment VI: Populate VI Ring\nPGSQL: Start Logger", "State(s) in (\"\")"=w436) -> ("States Out"=w435:string)  [unwired: 13 in]
      }
      frame "Macro: Exit" {
        # "Exit Macro\n(This is called once, when the VI exits)"
        n222 = Unbundle By Name(w444) -> ("Core.Close Panel on Exit?"=w443:bool)
        n223 = property on="OK" class="Bool (strict)"("Value"=FALSE ("Blinking")) -> ()  [unwired: 2 in, 2 out]
        n224 = Select(t="UI: Front Panel State >> Close", s=w443, f="") -> (s? t:f=w440:string)
        n225 = call <vilib>:"Add State(s) to Queue__jki_lib_state_machine.vi"("State(s) in (\"\")"=w440, "State(s) at Back (\"\")"="Data: Save Controls\nData: Cleanup\nExit") -> ("States Out"=w438:string)  [unwired: 13 in]
        n226 = call <vilib>:"Add State(s) to Queue__jki_lib_state_machine.vi"("State(s) in Front (\"\")"=w438, "State(s) in (\"\")"=w447) -> ("States Out"=w446:string)  [unwired: 13 in]
      }
      frame "Macro: Output" {
        n227 = case shown="False" "I'm Finished Taking Data!" {
          tunnel: [w462 _] -> w451
          frame False {
            n228 = local read "KH Addresses"() -> (w458:refnum<visa-resource-name>[])
            n229 = Empty Array?(array=w458) -> (empty?=w457:bool)
            n230 = Select(t="", s=w457, f="UI: SR Disable\nKH: set KH 0\nKH: set KH 1\nKH: set KH 2" ("State(s) in Front (\"\")")) -> (s? t:f=w459:string)
            n231 = call <vilib>:"Add State(s) to Queue__jki_lib_state_machine.vi"("State(s) in Front (\"\")"="Macro: Initialize Metadata" ("State(s) in Front (\"\")"), "State(s) in (\"\")"=w459, "State(s) at Back (\"\")"="Macro: Write Metadata" ("State(s) in Front (\"\")")) -> ("States Out"=w462:string)  [unwired: 12 in]
          }
          frame True {
          }
        }
        n232 = call <vilib>:"Add State(s) to Queue__jki_lib_state_machine.vi"("State(s) in Front (\"\")"=w451, "State(s) in (\"\")"=w454, "State(s) at Back (\"\")"="PGSQL: Write" ("State(s) in Front (\"\")")) -> ("States Out"=w453:string)  [unwired: 12 in]
      }
      frame "Macro: Initialize Metadata" {
        # "Do not put any code in this frame.\n(It is a separator no-op. You can make a copy of this frame to create a new Macro frame)"
        n233 = call <vilib>:"Add State(s) to Queue__jki_lib_state_machine.vi"("State(s) in Front (\"\")"="Metadata: Update Experiment Description\nMetadata: Update Wiring Configuration\nMetadata: Update KH\nMetadata: Build Path\nMetadata: Update Control Experiment Wire\n// Instruments: Load Classes\n// nstruments: Initialize KH" ("State(s) in Front (\"\")"), "State(s) in (\"\")"=w467) -> ("States Out"=w466:string)  [unwired: 13 in]
      }
      frame "Macro: Write Metadata" {
        # "Do not put any code in this frame.\n(It is a separator no-op. You can make a copy of this frame to create a new Macro frame)"
        n234 = call <vilib>:"Add State(s) to Queue__jki_lib_state_machine.vi"("State(s) in Front (\"\")"="Metadata: Update Comments\nMetadata: Write FGV\nMetadata: Write JSON" ("State(s) in Front (\"\")"), "State(s) in (\"\")"=w472) -> ("States Out"=w471:string)  [unwired: 13 in]
      }
      frame "---------- Metadata ----------" {
        n235 = call <vilib>:"Add State(s) to Queue__jki_lib_state_machine.vi"("State(s) in (\"\")"=w476) -> ("States Out"=w475:string)  [unwired: 14 in]
      }
      frame "Metadata: Update Experiment Description" {
        n236 = Concatenate Strings("Sample (SAXXXX)", "." ("string"), "Device (YYYYMMDD)") -> (w480:string)
        n237 = Bundle By Name(cluster=w484, "Experiment.Device"=w480, "Experiment.User"="Username", "Experiment.Device Description"="Description", "Experiment.Instrument"="Instrument") -> (w485:T24)
        n238 = call <vilib>:"Add State(s) to Queue__jki_lib_state_machine.vi"("State(s) in (\"\")"=w488) -> ("States Out"=w487:string)  [unwired: 14 in]
      }
      frame "Metadata: Update Wiring Configuration" {
        n239 = local read "Lockin"() -> (w497:T7)
        n240 = local read "non KH"() -> (w491:T10)
        n241 = local read "Lockin"() -> (w495:T7)
        n242 = Unbundle By Name(w491) -> ("Electrodes 2"=w490:string[], "Labels 2"=w489:u16[])
        n243 = Unbundle By Name(w495) -> ("Electrode Config"=w494:T6[])
        n244 = Unbundle By Name(w497) -> ("AI"=w492:u32[], "Electrode"=w493:string[], "Label"=w496:u16[])
        n245 = for {
          tunnel: w489 -> [w506] mode=indexing
          tunnel: [w505] -> w498 mode=indexing
          n246 = property on="Ring" class="Ring (strict)"() -> ("Strings []"=w507:string[])  [unwired: 2 in, 2 out]
          n247 = Index Array(array=w507, index=w506) -> (element=w505:string)
        }
        n248 = for {
          tunnel: w496 -> [w509] mode=indexing
          tunnel: [w508] -> w499 mode=indexing
          n249 = property on="Ring" class="Ring (strict)"() -> ("Strings []"=w510:string[])  [unwired: 2 in, 2 out]
          n250 = Index Array(array=w510, index=w509) -> (element=w508:string)
        }
        n251 = Bundle By Name(cluster=w500, "Wiring Configuration.Lockin Ch"=w492, "Wiring Configuration.KH.Electrodes"=w493, "Wiring Configuration.KH.Labels"=w499, "Wiring Configuration.not KH.Electrodes"=w490, "Wiring Configuration.not KH.Labels"=w498, "Lockin.Electrode Config"=w494) -> (w501:T24)
        n252 = call <vilib>:"Add State(s) to Queue__jki_lib_state_machine.vi"("State(s) in (\"\")"=w504) -> ("States Out"=w503:string)  [unwired: 14 in]
      }
      frame "Metadata: Update KH" {
        n253 = local read "KH"() -> (w525:T5)
        n254 = Unbundle By Name(w525) -> ("KH Gain"=w517:T3[], "KH Configuration"=w522:T2[], "KH Shunt Resistor"=w521:T4[], "KH #"=w514:u16[])
        n255 = Empty Array?(array=w514) -> (empty?=w515:bool)
        n256 = case shown="False" w515 {
          tunnel: [w538 w569] -> w524
          tunnel: w522 -> [w537 _]
          tunnel: w521 -> [w536 _]
          tunnel: [w535 w567] -> w520
          tunnel: w514 -> [w531 _]
          tunnel: [w534 w570] -> w519
          tunnel: [w533 w568] -> w518
          tunnel: w517 -> [w530 _]
          tunnel: w516 -> [w532 w570]
          tunnel: [w531 u16[] [] ("KH #")] -> w513
          frame False {
            n257 = Empty Array?(array=w530) -> (empty?=w529:bool)
            n258 = case shown="False" w529 {
              tunnel: [w553 w557] -> w538
              tunnel: w537 -> [w549 w559]
              tunnel: w536 -> [w548 w560]
              tunnel: [w547 w555] -> w535
              tunnel: [w546 w554] -> w534
              tunnel: [w545 w556] -> w533
              tunnel: w532 -> [w544 w554]
              tunnel: w530 -> [w540 w558]
              tunnel: w531 -> [w539 w561]
              frame False {
                n259 = call "Initialize KH Array.vi"("KH #"=w539, "Control in"=w540) -> ("Control out"=w552:variant)  [unwired: 9 in]
                n260 = call "Initialize KH Array.vi"("KH #"=w539, "Control in"=w549) -> ("Control out"=w551:variant)  [unwired: 9 in]
                n261 = call "Initialize KH Array.vi"("KH #"=w539, "Control in"=w548) -> ("Control out"=w550:variant)  [unwired: 9 in]
                n262 = Variant To Data(error in=w544, type=w540, Variant=w552) -> (data=w553:T3[], error out=w543:errorcluster)
                n263 = Variant To Data(error in=w544, type=w549, Variant=w551) -> (data=w545:T2[], error out=w542:errorcluster)
                n264 = Variant To Data(error in=w544, type=w548, Variant=w550) -> (data=w547:T4[], error out=w541:errorcluster)
                n265 = Merge Errors(w543, w542, w541) -> (w546:errorcluster)
              }
              frame True {
                n266 = Array Size(array=w561) -> (size(s)=w562:i32)
                n267 = Index Array(array=w559) -> (element=w564:T2)  [unwired: 1 in]
                n268 = Index Array(array=w560) -> (element=w563:T4)  [unwired: 1 in]
                n269 = Index Array(array=w558) -> (element=w565:T3)  [unwired: 1 in]
                n270 = Initialize Array(w565, w562) -> (w557:T3[])
                n271 = Initialize Array(w564, w562) -> (w556:T2[])
                n272 = Initialize Array(w563, w562) -> (w555:T4[])
              }
            }
          }
          frame True {
            w567 = T4[] [] items=["Open", "50 Ohms", "500 Ohms", "5k Ohms", "50k Ohms", "10M Ohm"] ("KH Shunt Resistor")
            w568 = T2[] [] items=["Ground", "SE+ (-gnd)", "SE- (+gnd)", "Differential"] ("KH Configuration")
            w569 = T3[] [] items=["1x", "10x", "100x", "1000x"] ("KH Gain")
          }
        }
        n273 = local read "KH All Buttons"() -> (w523:T8)
        n274 = Bundle By Name(cluster=w526, "KH All Buttons"=w523, "KH.KH Gain"=w524, "KH.KH Configuration"=w518, "KH.KH Shunt Resistor"=w520, "KH.KH #"=w513) -> (w512:T24)
        n275 = Unbundle By Name(w512) -> ("KH"=w511:T5)
        n276 = local write "KH"(w511) -> ()
        n277 = call <vilib>:"Add State(s) to Queue__jki_lib_state_machine.vi"("State(s) in (\"\")"=w528) -> ("States Out"=w527:string)  [unwired: 14 in]
      }
      frame "Metadata: Update AI" {
        n278 = local read "Lockin"() -> (w573:T7)
        n279 = Unbundle By Name(w573) -> ("Electrode"=w578:string[], "Label"=w583:u16[], "Electrode Config"=w582:T6[], "AI"=w575:u32[])
        n280 = Empty Array?(array=w575) -> (empty?=w576:bool)
        n281 = case shown="True" w576 {
          tunnel: [w597 string[] [] ("Electrode")] -> w584
          tunnel: w583 -> [w589 _]
          tunnel: w582 -> [w596 _]
          tunnel: [w595 w626] -> w581
          tunnel: w575 -> [w591 _]
          tunnel: [w590 w629] -> w580
          tunnel: [w594 u16[] [] ("Label")] -> w579
          tunnel: w578 -> [w592 _]
          tunnel: w577 -> [w593 w629]
          tunnel: [w591 u32[] [] ("AI")] -> w574
          frame False {
            n282 = Empty Array?(array=w589) -> (empty?=w588:bool)
            n283 = case shown="True" w588 {
              tunnel: [w612 w621] -> w597
              tunnel: w589 -> [w608 w622]
              tunnel: w596 -> [w607 w623]
              tunnel: [w606 w616] -> w595
              tunnel: [w605 w618] -> w594
              tunnel: w593 -> [w604 w613]
              tunnel: w592 -> [w600 w624]
              tunnel: w591 -> [w599 w615]
              tunnel: [w598 w613] -> w590
              frame False {
                n284 = call "Initialize KH Array.vi"("KH #"=w599, "Control in"=w600) -> ("Control out"=w611:variant)  [unwired: 9 in]
                n285 = call "Initialize KH Array.vi"("KH #"=w599, "Control in"=w608) -> ("Control out"=w610:variant)  [unwired: 9 in]
                n286 = call "Initialize KH Array.vi"("KH #"=w599, "Control in"=w607) -> ("Control out"=w609:variant)  [unwired: 9 in]
                n287 = Variant To Data(error in=w604, type=w600, Variant=w611) -> (data=w612:string[], error out=w603:errorcluster)
                n288 = Variant To Data(error in=w604, type=w608, Variant=w610) -> (data=w605:u16[], error out=w602:errorcluster)
                n289 = Variant To Data(error in=w604, type=w607, Variant=w609) -> (data=w606:T6[], error out=w601:errorcluster)
                n290 = Merge Errors(w603, w602, w601) -> (w598:errorcluster)
              }
              frame True {
                n291 = Array Size(array=w615) -> (size(s)=w614:i32)
                n292 = Index Array(array=w622) -> (element=w619:u16)  [unwired: 1 in]
                n293 = Index Array(array=w623) -> (element=w617:T6)  [unwired: 1 in]
                n294 = Index Array(array=w624) -> (element=w620:string)  [unwired: 1 in]
                n295 = Initialize Array(w620, w614) -> (w621:string[])
                n296 = Initialize Array(w619, w614) -> (w618:u16[])
                n297 = Initialize Array(w617, w614) -> (w616:T6[])
              }
            }
          }
          frame True {
            w626 = T6[] [] items=["Ground", "Current", "Voltage (SE)", "Voltage (Diff)", "Gate"] ("Electrode Config")
          }
        }
        n298 = Bundle By Name(cluster=w585, "Lockin.Electrode"=w584, "Lockin.Label"=w579, "Lockin.Electrode Config"=w581, "Lockin.AI"=w574) -> (w571:T24)
        n299 = Unbundle By Name(w571) -> ("Lockin"=w572:T7)
        n300 = local write "Lockin"(w572) -> ()
        n301 = call <vilib>:"Add State(s) to Queue__jki_lib_state_machine.vi"("State(s) in (\"\")"=w587) -> ("States Out"=w586:string)  [unwired: 14 in]
      }
      frame "Metadata: Build Path" {
        n302 = Unbundle By Name(w644) -> ("Experiment.Instrument"=w641:T9, "Experiment.Device"=w640:string)
        n303 = Format Into String(w641) -> (resulting string=w633:string)  [unwired: 3 in, 1 out]
        n304 = xnode "Match Regular Expression"("input string"=w633, "regular expression"=" \\(") -> ("before match"=w631:string, "error out"=w630:errorcluster)  [unwired: 4 in, 3 out]
        n305 = call <vilib>:"Clear Errors.vi"("error in (no error)"=w630) -> ()  [unwired: 5 in, 2 out]
        n306 = Build Path(base path="Default Path", name or relative path=w631) -> (appended path=w642:path)
        n307 = Build Path(base path=w642, name or relative path=w640) -> (appended path=w639:path)
        n308 = call <userlib>:"MGI Create Directory Chain.vi"("Error In"=w638, "File Presence (Auto Detect)"=MGI_Create_Directory_Chain_Behavior_Enum."Path Does Not Contain a File", "Path"=w639) -> ("Error Out"=w637:errorcluster, "Duplicate Path"=w635:path)  [unwired: 7 in]
        "Device Folder" <- w635
        n309 = Bundle By Name(cluster=w644, "Experiment.Device Path"=w635) -> (w643:T24)
        n310 = call <vilib>:"Add State(s) to Queue__jki_lib_state_machine.vi"("State(s) in (\"\")"=w646) -> ("States Out"=w645:string)  [unwired: 14 in]
      }
      frame "Metadata: Update Control Experiment Wire" {
        # "IS Control Experiment Class wire"
        # "Not on Control Experiment Class wire"
        n311 = Unbundle By Name(w765) -> ("C.E."=w763:refnum<class "Control Experiment.lvclass">, "Experiment"=w767:T19, "Wiring Configuration"=w766:T21)
        n312 = Bundle By Name(cluster=w763, "Experiment"=w767, "Wiring Configuration"=w766) -> (w761:refnum<class "Control Experiment.lvclass">)
        n313 = Bundle By Name(cluster=w765, "C.E."=w761) -> (w764:T24)
        n314 = call <vilib>:"Add State(s) to Queue__jki_lib_state_machine.vi"("State(s) in (\"\")"=w769) -> ("States Out"=w768:string)  [unwired: 14 in]
      }
      frame "Metadata: Update Comments" {
        # "error 63 occurs when\nthe lockin isn't running\nI think we can clear here?"
        n315 = Unbundle By Name(w780) -> ("C.E."=w776:refnum<class "Control Experiment.lvclass">)
        n316 = call "Generate Comments.vi"("error in (no error)"=w771, "Control Experiment"=w776) -> ("error out"=w773:errorcluster, "Control Experiment out"=w775:refnum<class "Control Experiment.lvclass">)  [unwired: 6 in, 1 out]
        n317 = call <vilib>:"Clear Errors.vi"("error in (no error)"=w773, "specific error code to clear (0: all)"=63) -> ("error out"=w772:errorcluster)  [unwired: 4 in, 1 out]
        n318 = call "Read Comments.vi"("error in (no error)"=w772, "Control Experiment in"=w775) -> ("error out"=w770:errorcluster, "Comments"=→"Comments":string, "Control Experiment out"=w777:refnum<class "Control Experiment.lvclass">)  [unwired: 7 in]
        n319 = Bundle By Name(cluster=w780, "C.E."=w777) -> (w779:T24)
        n320 = call <vilib>:"Add State(s) to Queue__jki_lib_state_machine.vi"("State(s) in (\"\")"=w782) -> ("States Out"=w781:string)  [unwired: 14 in]
      }
      frame "Metadata: Write FGV" {
        n321 = Unbundle By Name(w787) -> ("C.E."=w785:refnum<class "Control Experiment.lvclass">)
        n322 = call "Control Experiment FGV.vi"("Function"=enum16{"read", "write"}."write", "error in (no error)"=w783, "Control Experiment.lvclass"=w785) -> ("error out"=w784:errorcluster)  [unwired: 7 in, 1 out]
        n323 = call <vilib>:"Add State(s) to Queue__jki_lib_state_machine.vi"("State(s) in (\"\")"=w789) -> ("States Out"=w788:string)  [unwired: 14 in]
      }
      frame "Metadata: Read FGV" {
        n324 = call "Control Experiment FGV.vi"("Function"=enum16{"read", "write"}."read", "error in (no error)"=w793) -> ("error out"=w794:errorcluster, "Control Experiment.lvclass out"=w792:refnum<class "Control Experiment.lvclass">)  [unwired: 8 in]
        n325 = Bundle By Name(cluster=w790, "C.E."=w792) -> (w791:T24)
        n326 = call <vilib>:"Add State(s) to Queue__jki_lib_state_machine.vi"("State(s) in (\"\")"=w797) -> ("States Out"=w796:string)  [unwired: 14 in]
      }
      frame "Metadata: Write JSON" {
        w804 = T28 {"Device"={"Device"="", "User"="", "Time"="", "Computer Name"=""}, "Wiring"={"Lockin Ch"=[], "KH Electrodes"=[], "KH Labels"=[], "Other Electrodes"=[], "Other Labels"=[]}}  # Control Experiment JSON
        n327 = Unbundle By Name(w813) -> ("C.E."=w805:refnum<class "Control Experiment.lvclass">, "Experiment.Device"=w817:string, "Experiment.User"=w801:string)
        n328 = Unbundle By Name(w813) -> ("Lockin.AI"=w816:u32[], "Wiring Configuration.KH.Electrodes"=w815:string[], "Wiring Configuration.KH.Labels"=w814:string[], "Wiring Configuration.KH.Electrodes"=w811:string[], "Wiring Configuration.KH.Labels"=w810:string[])
        n329 = call "Get Date Time ISO.vi"() -> ("ISO 8601 date-time string"=w809:string)  [unwired: 9 in, 2 out]
        n330 = call "Get Computer Name.vi"() -> ("name"=w812:string)  [unwired: 10 in, 1 out]
        n331 = Bundle By Name(cluster=w804, "Device.Device"=w817, "Device.User"=w801, "Device.Time"=w809, "Device.Computer Name"=w812) -> (w803:T28)
        n332 = Bundle By Name(cluster=w803, "Wiring.Lockin Ch"=w816, "Wiring.KH Electrodes"=w815, "Wiring.KH Labels"=w814, "Wiring.Other Electrodes"=w811, "Wiring.Other Labels"=w810) -> (w800:T28)
        n333 = call "To JSON Text.vim"("Anything"=w800) -> ("<JSON>"=→"JSON String":string)  [unwired: 9 in, 1 out]
        n334 = call "Write Experiment Folder.vi"("error in (no error)"=w798, "Experiment Folder"="device", "Control Experiment in"=w805) -> ("error out"=w806:errorcluster, "Control Experiment out"=w807:refnum<class "Control Experiment.lvclass">)  [unwired: 7 in]
        n335 = call "Save JSON File.vi"("error in (no error)"=w806, "Data"=w800, "Control Experiment in"=w807) -> ("error out"=w808:errorcluster)  [unwired: 8 in]
        n336 = call <vilib>:"Add State(s) to Queue__jki_lib_state_machine.vi"("State(s) in (\"\")"=w819) -> ("States Out"=w818:string)  [unwired: 14 in]
      }
      frame "---------- KH ----------" {
        n337 = call <vilib>:"Add State(s) to Queue__jki_lib_state_machine.vi"("State(s) in (\"\")"=w823) -> ("States Out"=w822:string)  [unwired: 14 in]
      }
      frame "KH: set KH 0" {
        # "initialize the Channel Settings array"
        # "remove duplicates"
        n338 = local read "KH Addresses"() -> (w826:refnum<visa-resource-name>[])
        n339 = call "Remove Duplicates From 1D Array.vim"("array"=w826) -> ("array with duplicates removed"=w825:refnum<visa-resource-name>[])  [unwired: 10 in]
        n340 = local write "KH Addresses"(w825) -> ()
        n341 = Initialize Array(T15 {"Channel"=enum."Channel 1", "Gain"=enum."10x", "Bandwidth Filter"=enum."ON", "Shunt Resistor"=enum."50 Ohms", "Coupling"=enum."DC", "Input Config"=enum."Differential"} ("Channel Settings"), 8 ("dimension size")) -> (w832:T15[])
        n342 = Empty Array?(array=w825) -> (empty?=w827:bool)
        n343 = case shown="True" w827 {
          tunnel: w824 -> [w844 w859]
          tunnel: [w843 w859] -> w830
          tunnel: [w842 string[] []] -> w828
          tunnel: w825 -> [w841 _]
          frame False {
            n344 = for {
              tunnel: w841 -> [_] mode=indexing
              tunnel: [w848] -> w842 mode=concatenating
              tunnel: w844 -> [w847]
              tunnel: [w846] -> w843
              i -> [w850]
              n345 = call "Number to Letter.vi"("Number"=w850) -> ("Letter"=w849:string)
              n346 = for {
                N: 8 -> [_]
                tunnel: w849 -> [w855]
                tunnel: [w854] -> w848 mode=indexing
                tunnel: w847 -> [w853]
                tunnel: [w852] -> w846
                i -> [w857]
                n347 = Increment(x=w857) -> (x+1=w851:i32)
                n348 = Format Into String(format string="%s %d", error in=w853, w855, w851) -> (resulting string=w854:string, error out=w852:errorcluster)  [unwired: 1 in]
              }
            }
          }
          frame True {
          }
        }
        n349 = Array Size(array=w825) -> (size(s)=w835:i32)
        n350 = Bundle(w832) -> (w831:cluster{T15[]})  [unwired: 1 in]
        n351 = Initialize Array(w831, w835) -> (w836:cluster{T15[]}[])
        n352 = Bundle By Name(cluster=w838, "Channel Settings"=w836) -> (w837:T24)
        n353 = property on="Ring" class="Ring (strict)"(error in=w830, "Strings []"=w828) -> (error out=w829:errorcluster)  [unwired: 1 in, 1 out]
        n354 = call <vilib>:"Add State(s) to Queue__jki_lib_state_machine.vi"("State(s) in (\"\")"=w840) -> ("States Out"=w839:string)  [unwired: 14 in]
      }
      frame "KH: set KH 1" {
        n355 = Unbundle By Name(w871) -> ("Channel Settings"=w860:cluster{"Channel Setting":T22}[], "KH.KH #"=w873:u16[], "KH.KH Gain"=w876:T3[], "Lockin.Electrode Config"=w874:T6[], "KH.KH Shunt Resistor"=w875:T4[], "KH All Buttons"=w872:T8)
        n356 = local read "Bandwidth Filter"() -> (w861:bool)
        n357 = local read "DC Coupled"() -> (w862:bool)
        n358 = for {
          tunnel: w874 -> [w901] mode=indexing
          tunnel: w876 -> [w900] mode=indexing
          tunnel: w875 -> [w899] mode=indexing
          tunnel: w873 -> [w895] mode=indexing
          tunnel: [w904] -> w867 mode=indexing
          tunnel: w872 -> [w903]
          tunnel: [w902] -> w865 mode=indexing
          tunnel: [w898] -> w866 mode=indexing
          shift-right: [w891] -> w869
          shift-left: w860 -> [w892]
          tunnel: w862 -> [w887]
          tunnel: w861 -> [w882]
          n359 = property on="Ring" class="Ring (strict)"() -> ("Strings []"=w897:string[])  [unwired: 2 in, 2 out]
          n360 = case shown="\"No Selection\", Default" w903 {
            tunnel: w901 -> [w923 _ _]
            tunnel: [w928 Input_Configuration-Enum."Ground" ("Input Config") Input_Configuration-Enum."Differential" ("Input Config")] -> w898
            tunnel: w900 -> [w927 w946 w949]
            tunnel: [w926 w946 w949] -> w902
            tunnel: w899 -> [w925 _ _]
            tunnel: [w924 Shunt-Enum."Open" ("Shunt Resistor") w947] -> w904
            frame "No Selection", Default {
              n361 = case shown="\"Voltage (SE)\"" w923 {
                tunnel: [Input_Configuration-Enum."Ground" ("Input Config") Input_Configuration-Enum."Differential" ("Input Config") Input_Configuration-Enum."SE+ (-gnd)" ("Input Config") Input_Configuration-Enum."Differential" ("Input Config") Input_Configuration-Enum."Differential" ("Input Config")] -> w928
                tunnel: [Shunt-Enum."Open" ("Shunt Resistor") w932 Shunt-Enum."Open" ("Shunt Resistor") Shunt-Enum."Open" ("Shunt Resistor") Shunt-Enum."50k Ohms" ("Shunt Resistor")] -> w924
                tunnel: w927 -> [w929 w933 w936 w940 w942]
                tunnel: [w929 w933 w936 w940 w942] -> w926
                tunnel: w925 -> [_ w932 _ _ _]
                frame "Ground", Default {
                }
                frame "Current" {
                }
                frame "Voltage (SE)" {
                }
                frame "Voltage (Diff)" {
                }
                frame "Gate" {
                }
              }
            }
            frame "All Ground" {
            }
            frame "All Differential" {
              n362 = local read "Defualt Shunt Resistor"() -> (w947:T4)
            }
          }
          n363 = To Long Integer(number=w895) -> (32bit integer=w896:i32)
          n364 = Index Array(array=w897, index=w896) -> (element=w894:string)
          n365 = Select(t=Coupling-Enum."DC" ("Coupling"), s=w887, f=Coupling-Enum."AC" ("Coupling")) -> (s? t:f=w884:T18)
          n366 = Scan From String(format string="%s %d", input string=w894) -> (error out=w888:errorcluster, output 1=w890:string, output 2=w889:i32)  [unwired: 4 in, 2 out]
          n367 = Select(t=Filter-Enum."ON" ("Bandwidth Filter"), s=w882, f=Filter-Enum."OFF" ("Bandwidth Filter")) -> (s? t:f=w880:T17)
          n368 = case shown="No Error" w888 {
            tunnel: w904 -> [w921 _]
            tunnel: w902 -> [w920 _]
            tunnel: w898 -> [w919 _]
            tunnel: w892 -> [w911 w922]
            tunnel: [w910 w922] -> w891
            tunnel: w890 -> [w909 _]
            tunnel: w889 -> [w908 _]
            tunnel: w884 -> [w906 _]
            tunnel: w880 -> [w905 _]
            frame No Error {
              n369 = Decrement(x=w908) -> (x-1=w907:i32)
              n370 = call "Letter to Number.vi"("Letter"=w909) -> ("Number"=w912:i32)
              n371 = Index Array(array=w911, index=w912) -> (element=w917:cluster{"Channel Setting":T22})
              n372 = Unbundle(w917) -> ("Channel Setting"=w916:T22)
              n373 = Index Array(array=w916, index=w907) -> (element=w915:T15)
              n374 = Bundle By Name(cluster=w915, "Channel"=w907, "Gain"=w920, "Input Config"=w919, "Shunt Resistor"=w921, "Coupling"=w906, "Bandwidth Filter"=w905) -> (w914:T15)
              n375 = Replace Array Subset(array=w916, new element=w914, index=w907) -> (w918:T22)
              n376 = Bundle("Channel Setting"=w918) -> (w913:cluster{"Channel Setting":T22})  [unwired: 1 in]
              n377 = Replace Array Subset(array=w911, new element=w913, index=w912) -> (w910:cluster{"Channel Setting":T22}[])
            }
            frame Error {
            }
          }
        }
        n378 = local write "KH All Buttons"(T8."No Selection" ("KH All Buttons")) -> ()
        n379 = Bundle By Name(cluster=w871, "Channel Settings"=w869, "KH.KH Gain"=w865, "KH.KH Configuration"=w866, "KH.KH Shunt Resistor"=w867) -> (w877:T24)
        n380 = local read "KH"() -> (w868:T5)
        n381 = Bundle By Name(cluster=w868, "KH Gain"=w865, "KH Configuration"=w866, "KH Shunt Resistor"=w867) -> (w864:T5)
        n382 = local write "KH"(w864) -> ()
        n383 = call <vilib>:"Add State(s) to Queue__jki_lib_state_machine.vi"("State(s) in (\"\")"=w879) -> ("States Out"=w878:string)  [unwired: 14 in]
      }
      frame "KH: set KH 2" {
        n384 = Unbundle By Name(w959) -> ("Channel Settings"=w962:cluster{"Channel Setting":T22}[])
        n385 = Unbundle By Name(w959) -> ("C.E."=w957:refnum<class "Control Experiment.lvclass">)
        n386 = Unbundle By Name(w957) -> ("KH7008"=w956:refnum<class "Instrument.KH7008.lvclass">[])
        n387 = for {
          tunnel: w955 -> [w977]
          tunnel: [w969] -> w950
          tunnel: w962 -> [w976] mode=indexing
          tunnel: w956 -> [w975] mode=indexing
          tunnel: [w968] -> w960 mode=concatenating
          tunnel: [w967] -> w954 mode=indexing
          n388 = Unbundle(w976) -> ("Channel Setting"=w972:T22)
          n389 = call <userlib>:"Write Channel Setting.vi"("error in (no error)"=w977, "Channel Setting"=w972, "KH7008 in"=w975) -> ("error out"=w973:errorcluster, "KH7008 out"=w974:refnum<class "Instrument.KH7008.lvclass">)  [unwired: 7 in]
          n390 = call <userlib>:"KH Control.vi"("error in"=w973, "KH7008"=w974) -> ("error out"=w971:errorcluster, "KH7008.lvclass out"=w970:refnum<class "Instrument.KH7008.lvclass">)  [unwired: 8 in]
          n391 = call <userlib>:"Read Gain.vi"("error in (no error)"=w971, "KH7008 in"=w970) -> ("error out"=w969:errorcluster, "Gain"=w968:dbl[], "KH7008 out"=w967:refnum<class "Instrument.KH7008.lvclass">)  [unwired: 7 in]
        }
        n392 = local read "Gain"() -> (w961:dbl[])
        n393 = Bundle By Name(cluster=w957, "KH7008"=w954) -> (w958:refnum<class "Control Experiment.lvclass">)
        n394 = call "Multiply Gains.vi"("Other Gain"=w961, "Gain"=w960) -> ("Gain x Other Gain"=w952:dbl[])
        n395 = Unbundle By Name(w958) -> ("Lockin"=w953:refnum<class "Instrument.Lockin.lvclass">)
        n396 = call <userlib>:"setInputGain.vi"("error in (no error)"=w950, "InputGain"=w952, "Instrument.Lockin in"=w953) -> ("error out"=w951:errorcluster)  [unwired: 7 in, 1 out]
        n397 = Bundle By Name(cluster=w959, "C.E."=w958) -> (w964:T24)
        n398 = call <vilib>:"Clear Errors.vi"("error in (no error)"=w951) -> ("error out"=w963:errorcluster)  [unwired: 5 in, 1 out]
        n399 = call <vilib>:"Add State(s) to Queue__jki_lib_state_machine.vi"("State(s) in (\"\")"=w966) -> ("States Out"=w965:string)  [unwired: 14 in]
      }
      frame "---------- Instruments ----------" {
        n400 = call <vilib>:"Add State(s) to Queue__jki_lib_state_machine.vi"("State(s) in (\"\")"=w981) -> ("States Out"=w980:string)  [unwired: 14 in]
      }
      frame "Instruments: Load Classes" {
        n401 = Unbundle By Name(w989) -> ("C.E."=w987:refnum<class "Control Experiment.lvclass">)
        n402 = disable-structure shown="Enabled" {
          disable-tunnel: w987 -> [w997 w1001]
          disable-tunnel: [w996 w1000] -> w984
          disable-tunnel: [w995 w998] -> w986
          disable-tunnel: w985 -> [w994 w999]
          frame Disabled {
            n403 = call "Load Instrument Classes.vi"("error in (no error)"=w994, "Control Experiment.lvclass"=w997) -> ("error out"=w995:errorcluster, "Control Experiment out"=w996:refnum<class "Control Experiment.lvclass">)  [unwired: 8 in]
          }
          frame Enabled {
            n404 = call "Load Instrument Classes_New.vi"("error in (no error)"=w999, "C.E."=w1001) -> ("error out"=w998:errorcluster, "Control Experiment"=w1000:refnum<class "Control Experiment.lvclass">)  [unwired: 8 in]
          }
        }
        n405 = Unbundle By Name(w984) -> ("KH7008"=w982:refnum<class "Instrument.KH7008.lvclass">[])
        n406 = for {
          tunnel: [w992] -> w983 mode=indexing
          tunnel: w982 -> [_] mode=indexing
          i -> [w993]
          n407 = Number To Decimal String(number=w993) -> (decimal integer string=w992:string)  [unwired: 1 in]
        }
        n408 = Bundle By Name(cluster=w989, "C.E."=w984) -> (w988:T24)
        n409 = property on="KH Addresses" class="Arr (strict)"("Val(Sgnl)"=w983) -> ()  [unwired: 2 in, 2 out]
        n410 = call <vilib>:"Add State(s) to Queue__jki_lib_state_machine.vi"("State(s) in (\"\")"=w991) -> ("States Out"=w990:string)  [unwired: 14 in]
      }
      frame "---------- Experiment VI ----------" {
        n411 = call <vilib>:"Add State(s) to Queue__jki_lib_state_machine.vi"("State(s) in (\"\")"=w1005) -> ("States Out"=w1004:string)  [unwired: 14 in]
      }
      frame "Experiment VI: Populate VI Ring" {
        n412 = call <userlib>:"Current VIs Parent Directory__ogtk.vi"() -> ("Parent Directory (+ Relative)"=w1022:path)  [unwired: 5 in]
        n413 = call <userlib>:"String to 1D Array__ogtk.vi"("delimiter (Tab)"="\n", "string"="----Sweep Control----\nSweep Control.vi\nContinuous B Sweep.vi") -> ("Array of Strings"=w1008:string[])  [unwired: 9 in]
        n414 = call <userlib>:"String to 1D Array__ogtk.vi"("delimiter (Tab)"="\n", "string"="----Transport----\nIV.vi\nIV_Sweep.vi\nLockin_time.vi\nLockin_Vsg.vi\nLockin_sweep.vi\nLockin_AIWFM_time.vi\nTHz_TimeDelay.vi\nSweep_AIWFM_time.vi") -> ("Array of Strings"=w1007:string[])  [unwired: 9 in]
        n415 = Strip Path(path=w1022) -> (stripped path=w1019:path)  [unwired: 1 out]
        n416 = Build Path(base path=w1019, name or relative path="SweepControl") -> (appended path=w1018:path)
        n417 = Build Path(base path=w1019, name or relative path="Transport") -> (appended path=w1014:path)
        n418 = for {
          tunnel: w1018 -> [w1032]
          tunnel: w1008 -> [w1031] mode=indexing
          tunnel: [w1030] -> w1011 mode=indexing
          n419 = Build Path(base path=w1032, name or relative path=w1031) -> (appended path=w1030:path)
        }
        n420 = for {
          tunnel: w1014 -> [w1029]
          tunnel: w1007 -> [w1028] mode=indexing
          tunnel: [w1027] -> w1010 mode=indexing
          n421 = Build Path(base path=w1029, name or relative path=w1028) -> (appended path=w1027:path)
        }
        n422 = Build Array (concatenate)(w1011, w1010) -> (w1009:path[])
        n423 = Build Array (concatenate)(w1008, w1007) -> (w1006:string[])
        n424 = Bundle By Name(cluster=w1013, "VI paths"=w1009) -> (w1012:T24)
        n425 = property on="Ring" class="Ring (strict)"("Strings []"=w1006) -> ()  [unwired: 2 in, 2 out]
        n426 = call <vilib>:"Add State(s) to Queue__jki_lib_state_machine.vi"("State(s) in (\"\")"=w1026) -> ("States Out"=w1025:string)  [unwired: 14 in]
      }
      frame "Experiment VI: Open VI" {
        n427 = Unbundle By Name(w1038) -> ("VI paths"=w1037:path[])
        n428 = Index Array(array=w1037, index="Ring") -> (element=w1035:path)
        n429 = call "Open Experiment VI.vi"("error in (no error)"=w1034, "Path"=w1035) -> ("error out"=w1033:errorcluster)  [unwired: 9 in]
        n430 = call <vilib>:"Add State(s) to Queue__jki_lib_state_machine.vi"("State(s) in (\"\")"=w1040) -> ("States Out"=w1039:string)  [unwired: 14 in]
      }
      frame "Experiment VI: Open Lockin" {
        n431 = call "Open Lockin.vi"("error in (no error)"=w1042) -> ("error out"=w1041:errorcluster)  [unwired: 10 in]
        n432 = call <vilib>:"Add State(s) to Queue__jki_lib_state_machine.vi"("State(s) in (\"\")"=w1045) -> ("States Out"=w1044:string)  [unwired: 14 in]
      }
      frame "---------- PGSQL ----------" {
        n433 = call <vilib>:"Add State(s) to Queue__jki_lib_state_machine.vi"("State(s) in (\"\")"=w1049) -> ("States Out"=w1048:string)  [unwired: 14 in]
      }
      frame "PGSQL: Start Logger" {
        n434 = Unbundle By Name(w1051) -> ("Logger"=w1056:refnum<class "Logger.PGSQL.lvclass">)
        n435 = call <vilib>:"Create.vi"("error in (no error)"=w1053, "SMO"=w1056) -> ("error out"=w1055:errorcluster, "SMO out"=w1057:refnum<class "Logger.PGSQL.lvclass">)  [unwired: 7 in, 1 out]
        n436 = call <vilib>:"Start.vi"("error in (no error)"=w1055, "SMO"=w1057) -> ("error out"=w1052:errorcluster, "SMO out"=w1054:refnum<class "Logger.PGSQL.lvclass">)  [unwired: 8 in]
        n437 = Bundle By Name(cluster=w1051, "Logger"=w1054) -> (w1050:T24)
        n438 = call <vilib>:"Add State(s) to Queue__jki_lib_state_machine.vi"("State(s) in (\"\")"=w1059) -> ("States Out"=w1058:string)  [unwired: 14 in]
      }
      frame "PGSQL: Write" {
        w1071 = "" ("f")
        n439 = Unbundle By Name(w1075) -> ("Logger"=w1069:refnum<class "Logger.PGSQL.lvclass">, "Experiment.Instrument"=w1060:T9, "Experiment.Device"=w1074:string, "Experiment.User"=w1073:string)
        n440 = local read "I'm Finished Taking Data!"() -> (w1072:bool)
        n441 = Not(x=w1072) -> (.not. x?=w1070:bool)
        n442 = call "Device and User PGSQL Paths.vi"("instrument"=w1060) -> ("User Path"=w1062:string, "Device Path"=w1068:string)  [unwired: 5 in]
        n443 = Select(t=w1074, s=w1070, f=w1071) -> (s? t:f=w1067:string)
        n444 = Select(t=w1073, s=w1070, f=w1071) -> (s? t:f=w1061:string)
        n445 = call <userlib>:"Logger.PGSQL.WriteVariable.vi"("error in (no error)"=w1065, "Data"=w1067, "Address"=w1068, "Logger"=w1069) -> ("error out"=w1064:errorcluster, "Logger out"=w1066:refnum<class "Logger.PGSQL.lvclass">)  [unwired: 6 in]
        n446 = call <userlib>:"Logger.PGSQL.WriteVariable.vi"("error in (no error)"=w1064, "Data"=w1061, "Address"=w1062, "Logger"=w1066) -> ("error out"=w1063:errorcluster)  [unwired: 6 in, 1 out]
        n447 = call <vilib>:"Add State(s) to Queue__jki_lib_state_machine.vi"("State(s) in (\"\")"=w1077) -> ("States Out"=w1076:string)  [unwired: 14 in]
      }
    }
  }
  "Error Out" <- w2
  n448 = Unbundle By Name(w6) -> ("C.E."=→"Control Experiment":refnum<class "Control Experiment.lvclass">)
